vi "ziExample-HF2-ImpedanceSweep.vi"() -> ()   [LabVIEW 2009]
doc: "Control a Zurich instrument device via the LabOne Labview API. \nRequirements: Zurich Instruments HF2 (HF2IS or HF2LI-MF ).\nThis example uses the API functions to perform a frequency sweep and measure the impedance. \n\n© Zurich Instruments AG, www.zhinst.com"
uses:
  <instrlib>/Zurich Instruments LabOne/Public/Utility/Impedance/ziTypeCalib.ctl
  <instrlib>/Zurich Instruments LabOne/Public/Utility/Impedance/ziTypeCalibModel.ctl
  <instrlib>/Zurich Instruments LabOne/Public/Utility/Impedance/ziTypeImpedanceEqCircModel.ctl
  <vilib>/Utility/file.llb/Write To Spreadsheet File (DBL).vi
  <instrlib>/Zurich Instruments LabOne/Zurich Instruments LabOne.lvlib
panel:
  out "Selected Device":string
  in  "Address":string="DEV"
  out "output cluster":T1
  out "Cmd":enum16{"Idle", "Calibrate", "Measure"}(ring)
  in  "Log Sweep":bool
  in  "Voltage Gain 2":dbl=1.0 caption="Volt. Gain"
  in  "Voltage Gain":dbl=1.0 caption="Volt. Gain"
  in  "Shunt Resistor":dbl=10.0 caption="Shunt Res"
  out "cal_types":cluster{string[], bool[]}[](array[cluster])=[{["R (Ohms)", " ", " "], [TRUE, FALSE, FALSE]}, {["C (F)", " ", " "], [TRUE, FALSE, FALSE]}, {["L (H)", " ", " "], [TRUE, FALSE, FALSE]}, {["R (Ohms)", "C (F)\n ", " "], [TRUE, TRUE, FALSE]}]
  in  "PreampChannel":dbl(ring) items=["1", "2"]
  in  "Iz Demod":i32 caption="Demod"
  out "Point":i32=10 caption="Point (#)"
  in  "Iz ZCtrl":dbl(ring) items=["1", "2"]
  in  "Vz ZCtrl":dbl(ring)=1.0 caption="CA ZCtrl" items=["1", "2"]
  in  "Vz Demod":i32=3
  in  "Vz Mode":u16(ring)=1 items=["From Sig Out", "Signal Input", "HF2CA"]
  in  "Iz Mode":u16(ring)=2 items=["HF2TA", "HF2CA", "Int. Shunt", "Ext. Shunt"]
  in  "Tab Control":enum32{"Measurement", "Calibration"}(tab)
  in  "CalApply":bool
  out "Vz: Amp":T2(graph)
  out "Vz: Theta":T2(graph)
  out "C (F)":cluster{"Output":dbl[], dbl[]}(graph)={"Output"=[1000000.0, 1394950.79396242, 1945887.7175763901, 2714417.616594907, 3786479.009414645, 5281951.900505007, 7368062.997280774, 10278085.328021964, 14337423.28873774, 20000000.000000004], []}
  out "Iz (Arms)":cluster{"Output":dbl[], dbl[]}(graph)={"Output"=[1000000.0, 1394950.79396242, 1945887.7175763901, 2714417.616594907, 3786479.009414645, 5281951.900505007, 7368062.997280774, 10278085.328021964, 14337423.28873774, 20000000.000000004], []}
  out "Phase(I) (deg)":cluster{"Output":dbl[], dbl[]}(graph)={"Output"=[1000000.0, 1394950.79396242, 1945887.7175763901, 2714417.616594907, 3786479.009414645, 5281951.900505007, 7368062.997280774, 10278085.328021964, 14337423.28873774, 20000000.000000004], []}
  out "Raw Theta":cluster{dbl[], dbl[]}[](graph)=[{[1000000.0, 1394950.79396242, 1945887.7175763901, 2714417.616594907, 3786479.009414645, 5281951.900505007, 7368062.997280774, 10278085.328021964, 14337423.28873774, 20000000.000000004], [-2.125111002254364, -2.9180042427061874, -4.0042554137336674, -5.49361529933484, -7.575470258948731, -10.468749002646796, -14.656165010490133, -20.60629193272774, -29.257773273212596, -42.298319052614715]}, {[1000000.0, 1394950.79396242, 1945887.7175763901, 2714417.616594907, 3786479.009414645, 5281951.900505007, 7368062.997280774, 10278085.328021964, 14337423.28873774, 20000000.000000004], [-1.9735738261703217, -2.706927178851299, -3.6423625337918537, -4.9685737214455274, -6.862030199908028, -9.497652129209763, -13.252753090507843, -18.663185630274253, -26.628128185477088, -38.88126041886271]}, {[1000000.0, 1394950.79396242, 1945887.7175763901, 2714417.616594907, 3786479.009414645, 5281951.900505007, 7368062.997280774, 10278085.328021964, 14337423.28873774, 20000000.000000004], [0.15153717608404205, 0.21107706385488845, 0.36189287994181374, 0.5250415778893123, 0.7134400590407033, 0.9710968734370322, 1.4034119199822896, 1.9431063024534865, 2.6296450877355078, 3.4170586337520064]}]
  in  "Sweep":bool
  out "Raw Voltage":cluster{dbl[], dbl[]}[](graph)=[{[1000000.0, 1394950.79396242, 1945887.7175763901, 2714417.616594907, 3786479.009414645, 5281951.900505007, 7368062.997280774, 10278085.328021964, 14337423.28873774, 20000000.000000004], [0.023378137138417795, 0.023352635540891502, 0.02333887818292926, 0.023325702784780588, 0.023293571728526332, 0.02327435029470388, 0.023266098096908466, 0.023207676828308578, 0.023122435350856608, 0.022822802880295735]}, {[1000000.0, 1394950.79396242, 1945887.7175763901, 2714417.616594907, 3786479.009414645, 5281951.900505007, 7368062.997280774, 10278085.328021964, 14337423.28873774, 20000000.000000004], [0.011672305817526927, 0.011652162485173598, 0.01164073320249789, 0.011628802299049338, 0.011618688750611094, 0.011628538960158322, 0.011638988104010175, 0.011664869376525768, 0.011693607080250431, 0.011687890332164705]}]
  in  "SaveData":bool
  out "R (ohm)":cluster{"Output":dbl[], dbl[]}(graph)={"Output"=[1000000.0, 1394950.79396242, 1945887.7175763901, 2714417.616594907, 3786479.009414645, 5281951.900505007, 7368062.997280774, 10278085.328021964, 14337423.28873774, 20000000.000000004], []}
  out "cmp1":dbl caption="|Z| (Ohm)" format="%_5p"
  out "cmp2":dbl caption="Phi (deg)" format="%_5p"
  out "Extrapolated":bool
  in  "Unit Sel":T3=enum."|Z|, Phi"
  in  "CalibPlot":bool
  in  "Calibrate":bool
  out "Calibration Theta (deg)":T4(graph)
  in  "SaveCalib":bool
  in  "LoadCalib":bool
  in  "Calib Container":T5(array[cluster])=[{"Ref Label"="49.9", "Ref ID"=1, "Ref_Z"=[49.9+0.0i], "Meas_Z"=[100.0, 50.23729761312895, 2.121440574135451e-05, 101.32221485214248, 50.24456461049771, -2.6268567656583807e-05, 102.66191222543722, 50.24501670088856, -6.196503568242303e-05, 104.01932327637543, 50.2446244843673, -5.713301200835168e-05, 105.39468221783378, 50.24416304621723, -5.367452327358224e-05, 106.78822635948634, 50.24524269734806, -5.876089144636414e-05, 108.200196148751, 50.246354974997864, -6.364545386253118e-05, 109.63083521227709, 50.24671592753094, -6.067752029835185e-05, 111.08039039798167, 50.24580811649929, -6.479615187070807e-05, 112.54911181764163, 50.247002863074755, -5.827912157445999e-05, 114.03725289004895, 50.24804205709008, -5.481035794834855e-05, 115.54507038473645, 50.24917669390061, -5.335595986182831e-05, 117.07282446628192, 50.246949394358616, -7.292141020097264e-05, 118.6207787391978, 50.24882796722916, -6.750797590795425e-05, 120.18920029341454, 50.247846007499454, -5.7847329975082594e-05, 121.77835975036535, 50.24845718404789, -4.293736826430601e-05, 123.38853130968018, 50.248343510682076, -6.311796069229001e-05, 125.01999279649725, 50.249183273366306, -7.942521692783592e-05, 126.6730257094, 50.24772866257277, -7.427869435562275e-05, 128.34791526898795, 50.2476915178063, -7.601733111173622e-05, 130.04495046708976, 50.245533237900865, -5.583774108413694e-05, 131.76442411662694, 50.24753693734964, -7.248396684417506e-05, 133.506632902137, 50.24762342206959, -8.020141468398587e-05, 135.2718774309644, 50.24738695570386, -8.318556929612295e-05, 137.06046228512858, 50.249066459043476, -7.02076550143384e-05, 138.8726960738777, 50.24848771373767, -8.1871266738444e-05, 140.7088914869372, 50.24868744189634, -7.362994992315661e-05, 142.56936534846253, 50.25014472956201, -6.385281326676391e-05, 144.4544386717052, 50.25079362150357, -8.842270680225136e-05, 146.36443671440153, 50.24791809805706, -7.87625706591446e-05, 148.29968903489402, 50.24918621159905, -1.4247528741100358e-05, 150.26052954899453, 50.24700324146568, 2.4328293243222397e-05, 152.24729658759927, 50.24742659667306, -8.207366957398373e-05, 154.2603329550659, 50.24824371666022, -9.25027016414374e-05, 156.29998598836224, 50.24936659001939, -7.856629604557065e-05, 158.366607616997, 50.247703627076696, -8.101461803112264e-05, 160.46055442374313, 50.24847444541704, -8.360916870339348e-05, 162.58218770616404, 50.24684762067942, -8.42162391563758e-05, 164.7318735389531, 50.247774868237755, -9.143276825460823e-05, 166.90998283709771, 50.24751479542865, -9.083054064933006e-05, 169.11689141987827, 50.24687854762921, -8.032930312132663e-05, 171.3529800757136, 50.245454152632874, -0.0001002428490940411, 173.61863462786343, 50.24374595275946, -9.273543582695971e-05, 175.91424600100004, 50.24399446647822, -8.930879950739245e-05, 178.2402102886597, 50.24463642269349, -8.9468508221365e-05, 180.59692882158637, 50.24433860831839, -0.00010562198902211549, 182.98480823697858, 50.24378130866547, -9.00820622436489e-05, 185.40426054865233, 50.24277723345728, -8.794795152361801e-05, 187.85570321813157, 50.24262820801012, -9.394497153337508e-05, 190.3395592266784, 50.24087696315062, -9.303875911910995e-05, 192.8562571482761, 50.240156107300876, -0.00010294840330862538, 195.4062312235767, 50.23942030425392, -0.00010216217241291718, 197.9899214348267, 50.24028214134422, -7.679878497665776e-05, 200.60777358178322, 50.24331740451916, -4.877843237779148e-05, 203.2602393586339, 50.237629543368605, -0.00014412323110584457, 205.94777643193413, 50.237242860989426, -0.00010368709185469055, 208.67084851957435, 50.23652108204443, -0.00010531426997736317, 211.42992547079191, 50.237714097600175, -0.00011317987522256575, 214.2254833472405, 50.23871809659533, -0.00010741394236277056, 217.05800450513172, 50.23657830717324, -0.00012093921870647237, 219.9279776784627, 50.23688431881305, -0.00011039496993179517, 222.83589806334393, 50.237727239145066, -0.00011666302857080836, 225.78226740344255, 50.237920119171335, -0.0001132697762300105, 228.7675940765549, 50.23898063887997, -0.00011842913699133826, 231.79239318232413, 50.23695928588504, -0.00012264440046028195, 234.85718663111734, 50.236623190031594, -0.00012009527011622733, 237.96250323407796, 50.23849833701747, -0.0001160793104080237, 241.10887879436896, 50.23885709351022, -0.00011923738836989553, 244.29685619962234, 50.23875634780288, -0.00012605945243077108, 247.5269855156109, 50.235412702723224, -0.00014489924302107032, 250.79982408115887, 50.234219003536516, -0.00013231674153141434, 254.11593660430717, 50.235578849530135, -0.00013377463756983191, 257.4758952597503, 50.235443222241436, -0.0001349608674113157, 260.88027978756156, 50.236126095861316, -0.00013179524516250768, 264.32967759322355, 50.23542562417865, -0.00013391534137439175, 267.82468384898175, 50.23625165516228, -0.00014298573817566227, 271.3659015965364, 50.23690727788916, -0.00015680990817982095, 274.95394185109643, 50.23658453903392, -0.0001400935583827526, 278.5894237068025, 50.2379820454398, -0.00015305640734792158, 282.2729744435523, 50.23779555499338, -0.0001454244383816006, 286.005229635229, 50.23633598000316, -0.00015199925922369304, 289.7868332593705, 50.23750893219329, -0.0001422943141655904, 293.618437808279, 50.23826807223343, -0.00014498739479441598, 297.5007044016091, 50.24257243523222, -0.0002208232263127257, 301.43430290043534, 50.233676447783004, -8.696126824219892e-05, 305.4199120228374, 50.237018744070234, -0.00015812075664359103, 309.4582194610035, 50.23840482558237, -0.0001421567736495156, 313.54992199989294, 50.23720959526779, -0.00016391008918537842, 317.69572563745635, 50.238882279353724, -0.0001747339577064879, 321.89634570645694, 50.23817479484266, -0.00016711708268028609, 326.1525069978913, 50.23794493404207, -0.00016987432226198176, 330.4649438860528, 50.23942799702911, -0.00018019706189285748, 334.8344004552382, 50.239504175654254, -0.00017134177816558637, 339.2616306281399, 50.23854749803337, -0.00018134810219163985, 343.7473982959256, 50.239863616591016, -0.00018691169923698288, 348.29247745004807, 50.24004166104534, -0.00022403392716366483, 352.89765231578724, 50.24138303687455, -0.0001633680357283863, 357.5637174875691, 50.24132555893579, -0.00018109919688103212, 362.29147806606215, 50.24012695672146, -0.00019152917023744354, 367.08174979709855, 50.24048343767394, -0.00019087901930413202, 371.9353592124199, 50.23935600994191, -0.00018980468877723996, 376.8531437722964, 50.23945619593062, -0.00019207175954793134, 381.8359520100192, 50.23941024460613, -0.00019504023060529945, 386.8846436783157, 50.24004177721329, -0.00019049824526780213, 392.0000898976885, 50.23936798873412, -0.00022604853872247393, 397.183173306728, 50.23924109279576, -0.00013131812397570967, 402.4347882144, 50.23465524046287, -0.00016094847498827718, 407.7558407543593, 50.237935578787884, -0.00023442906566915965, 413.1472490412919, 50.23754191590512, -0.0002241082550303329, 418.609943329334, 50.23758477571322, -0.00020745270535459898, 424.14486617257967, 50.23844955352966, -0.00022638680937830992, 429.7529725877134, 50.23819284665975, -0.0002199711780855827, 435.4352302187919, 50.23848807847116, -0.00021746871784881117, 441.1926195042056, 50.23752737389911, -0.0002347905781568576, 447.0261338458467, 50.23723095212465, -0.00023695481260912191, 452.93677978051477, 50.237967943967085, -0.00023321305655591763, 458.9255771535886, 50.237296399116545, -0.00023583442488857333, 464.993559294994, 50.23819243539614, -0.00022819779420788495, 471.14177319749837, 50.23821404307303, -0.00023657243075930968, 477.37127969736315, 50.238454297395336, -0.0002564686351001599, 483.6831536573843, 50.23949055231677, -0.00025662562140457847, 490.0784841523534, 50.23963343470409, -0.00026991681507969946, 496.55837465697056, 50.24006446546527, -0.00019542383543565305, 503.1239432362423, 50.24006149866944, -0.00019263605772786905, 509.7763227383968, 50.241541900367416, -0.0002650210010511269, 516.5166609903497, 50.24204575422077, -0.0002680894028589533, 523.3461209957545, 50.24192028206883, -0.0002595992513746522, 530.265881135672, 50.24243515517191, -0.0002693038142289864, 537.2771353718921, 50.24194685410137, -0.00028033155549634563, 544.3810934529448, 50.243606525411785, -0.0002760762107079244, 551.5789811228353, 50.242950307895605, -0.0002691784388977296, 558.8720403325376, 50.24270972720745, -0.00028235834370080135, 566.2615294542862, 50.242641696523165, -0.0002813688997713343, 573.7487234987, 50.24297072057299, -0.0002886415178501039, 581.3349143347776, 50.24155585194577, -0.00028813043222880976, 589.0214109128019, 50.241512211068226, -0.00030399847025470696, 596.8095394901901, 50.246494416914686, -0.00030000047211699543, 604.7006438603325, 50.2411127859893, -0.00032191837745573814, 612.6960855844551, 50.24388358908722, -0.00032557214682823766, 620.7972442265484, 50.24425956315106, -0.0003281739605617717, 629.0055175914031, 50.24376088901165, -0.0003249400740398162, 637.3223219657923, 50.24400596262748, -0.00032628094469877784, 645.7490923628433, 50.243892945867564, -0.0003149332196067413, 654.2872827696401, 50.244689616316684, -0.0003224844489783764, 662.9383663980998, 50.24448603801334, -0.0003296492473939034, 671.7038359391662, 50.24385175285881, -0.00034531896154369097, 680.5852038203647, 50.2433017558709, -0.00035427140131504394, 689.5840024667617, 50.24254002402706, -0.000351718688616745, 698.7017845653758, 50.24426996580821, -0.00034292404995620675, 707.9401233330838, 50.242294710892395, -0.0003511291528132747, 717.3006127880695, 50.24320044074088, -0.000357591418540799, 726.7848680248625, 50.24384831032141, -0.0003581451947597097, 736.3945254930113, 50.24411746233949, -0.0003624322702113084, 746.1312432794441, 50.245400714741756, -0.0003768273094781495, 755.9967013945603, 50.24460116850206, -0.00038515303493329487, 765.9926020621064, 50.24386501335661, -0.0004014769252018121, 776.1206700128843, 50.24343741635483, -0.0003850526766427019, 786.3826527823423, 50.242386569716956, -0.0003944547277776726, 796.7803210121025, 50.24231847213171, -0.0004083242796739145, 807.315468755473, 50.24148533783557, -0.0004069646661488162, 817.9899137870017, 50.24304518383028, -0.0004043264799102493, 828.8054979161209, 50.24321435653486, -0.0004082179233760825, 839.7640873049413, 50.242901199777, -0.0004233529907266768, 850.867572790246, 50.24335396992659, -0.00041494558073980244, 862.1178702097428, 50.24285017263916, -0.0004250528520568761, 873.5169207326305, 50.24421089963702, -0.00044036646096422516, 885.066691194535, 50.243906111732, -0.0004455635019504344, 896.7691744368752, 50.243115112962, -0.00044548362054011836, 908.6263896507152, 50.241847736633005, -0.0004546709589164505, 920.6403827251629, 50.242469741042036, -0.000469671885646098, 932.8132266003764, 50.24200716387695, -0.0004755603159924677, 945.1470216252361, 50.242235520185325, -0.00046569926345137625, 957.6438959197473, 50.24228264021354, -0.0004560626191996769, 970.3060057422341, 50.241726115331836, -0.0004693435526159942, 983.1355358613883, 50.24250104649113, -0.000469173165346523, 996.1346999332383, 50.242280221489466, -0.0004941911752693712, 1009.3057408831005, 50.241041961032785, -0.0004972471672201722, 1022.6509312925836, 50.24065192046913, -0.0005048544802369564, 1036.1725737917075, 50.240705322833705, -0.0005120142985370826, 1049.8730014562084, 50.2409880560542, -0.0005185151977316893, 1063.7545782100965, 50.24100716912316, -0.0005256851906550238, 1077.819699233536, 50.23957008666112, -0.0005233075405538072, 1092.0707913761194, 50.24066642423129, -0.0005667882309460218, 1106.5103135756042, 50.24028373804092, -0.0005886985493355609, 1121.1407572821893, 50.23984181544734, -0.0005416423273569886, 1135.964646888397, 50.23901186463722, -0.0005469432103160592, 1150.9845401646432, 50.23992880526662, -0.000563876372453988, 1166.2030287005641, 50.239552851083815, -0.0005613410906528647, 1181.6227383521784, 50.239819261152476, -0.00055276476146632, 1197.2463296949636, 50.23718308658164, -0.00059155470497235, 1213.0764984829211, 50.23703227282794, -0.0005639536793866361, 1229.1159761137123, 50.23720604014747, -0.0005828010566710451, 1245.367530099944, 50.2376316294328, -0.000605006915033908, 1261.8339645466854, 50.23706673631338, -0.000605622450206069, 1278.5181206353, 50.23635119432776, -0.0006167725116433101, 1295.422877113673, 50.23539548733378, -0.0006297581002267215, 1312.5511507929214, 50.236467808934, -0.0006640770731730505, 1329.9058970506724, 50.23718535641903, -0.0006493956219717666, 1347.490110340995, 50.23597810259524, -0.0006575973144651183, 1365.3068247110748, 50.23612858584978, -0.0006552481232708702, 1383.3591143247195, 50.234825849623896, -0.0006571084498600002, 1401.6500939927878, 50.23411209669829, -0.0006556132494747068, 1420.1829197106294, 50.237073548758374, -0.0006957885218835113, 1438.960789202634, 50.23609605743348, -0.0006716559593610621, 1457.986942473978, 50.23655785267992, -0.0006847225644928291, 1477.2646623696671, 50.2367756747552, -0.0007089642012018262, 1496.7972751409714, 50.23461986858555, -0.0007235796678223535, 1516.5881510193492, 50.23777867946216, -0.0007067022205569458, 1536.64070479796, 50.23594013773257, -0.0007350784198242394, 1556.9583964208657, 50.23548638970917, -0.0007277415031621394, 1577.5447315800218, 50.23577058239413, -0.0007365114353948249, 1598.403262320164, 50.234764438996656, -0.0007358475139249357, 1619.5375876516912, 50.23451293620078, -0.0007669913805915337, 1640.951354171652, 50.2342973593145, -0.0007672584900687068, 1662.6482566929444, 50.234877383456855, -0.0007719410590508477, 1684.6320388818249, 50.23479457558916, -0.0007975876224606731, 1706.9064939038728, 50.23411424828983, -0.0007839190573285075, 1729.4754650784525, 50.23335239475232, -0.0008236858193597738, 1752.342846541882, 50.233956339633075, -0.0008219820643363365, 1775.5125839193133, 50.23267459889144, -0.0008248354222896179, 1798.988675005555, 50.23209385202891, -0.0008258347765294869, 1822.7751704548377, 50.23233597449878, -0.0008402376745349847, 1846.8761744797591, 50.232063575711535, -0.0008434684927485383, 1871.2958455594094, 50.23226069711804, -0.0008495184625211668, 1896.038397156923, 50.231264787120935, -0.000856226416158429, 1921.1080984464543, 50.23071209814313, -0.0008779962269724759, 1946.5092750498272, 50.23171826210217, -0.00089508111780188, 1972.246309782865, 50.22893609855841, -0.0009023291566507657, 1998.3236434116482, 50.229671960519234, -0.0009343517002818267, 2024.7457754187096, 50.228264240727206, -0.000923053626219264, 2051.517264779425, 50.22793750616886, -0.0009217625619728219, 2078.642730748604, 50.22715368622507, -0.0009448586201383313, 2106.1268536575444, 50.22981498597677, -0.0009480664328276984, 2133.9743757215633, 50.22753294140639, -0.00097696946339409, 2162.1901018582707, 50.229106040780856, -0.0009795278451825758, 2190.7789005165932, 50.22925952739951, -0.000964143533363214, 2219.74570451683, 50.22913336910716, -0.000999664726629083, 2249.095511901744, 50.22888765446308, -0.0009929226999867554, 2278.833386798981, 50.229156943383416, -0.0010356702222864209, 2308.9644602948165, 50.2275218915404, -0.001023076393648231, 2339.493931319528, 50.22746275489175, -0.0010120517700893503, 2370.427067544405, 50.2281958047674, -0.001026785817893122, 2401.769206290685, 50.22815050358506, -0.0010515565170741634, 2433.5257554504424, 50.22735832444823, -0.0010546438729483237, 2465.702194419723, 50.2270696074257, -0.0010765612187811227, 2498.3040750439413, 50.22765197797887, -0.0011118182352407738, 2531.337022575856, 50.2276471510043, -0.001101844497572114, 2564.8067366461323, 50.22721822901245, -0.0011337329910801146, 2598.718992246821, 50.22720426028747, -0.001122893143006475, 2633.0796407277535, 50.22443066210692, -0.00116261967665977, 2667.894610806198, 50.226871660032785, -0.0011483106083631292, 2703.1699095897843, 50.22526274815143, -0.0011507616972477122, 2738.9116236130294, 50.223806897500516, -0.001173247560470509, 2775.125919887495, 50.22634928448615, -0.0011913188342702536, 2811.819046965906, 50.2258071872988, -0.0011988830826533568, 2848.9973360202575, 50.22419364937601, -0.0012148498702072607, 2886.667201934264, 50.22282751934193, -0.0012123971632495361, 2924.835144410162, 50.222894099248904, -0.0012330284118999585, 2963.507749090239, 50.22246247680122, -0.001264311966019769, 3002.6916886931003, 50.221090275797124, -0.0012558228823002556, 3042.3937241650515, 50.22071885090921, -0.0012853768065090344, 3082.6207058466093, 50.221689332713005, -0.0012939793355571283, 3123.379574654536, 50.219118508740856, -0.0012900490004014427, 3164.6773632793997, 50.22018200020054, -0.001321423076319436, 3206.521197399074, 50.219804467487094, -0.0013217581465878262, 3248.9182969081785, 50.21896416346328, -0.0013519130644718818, 3291.8759771638765, 50.21723415283566, -0.0013394520641220394, 3335.401650248044, 50.21907848822479, -0.0013708606750503596, 3379.502826246233, 50.217898207990075, -0.001378802620359021, 3424.187114543432, 50.21712744965305, -0.0013947676225755856, 3469.462225137078, 50.21626045719793, -0.0014316210807793785, 3515.3359699673097, 50.21657172729146, -0.0014384263510618701, 3561.816264264928, 50.21680400626807, -0.0014298789475400897, 3608.911127917062, 50.21542751168883, -0.0014498958934021917, 3656.628686851008, 50.21531737343841, -0.0014561937888761822, 3704.9771744362506, 50.21600817244085, -0.001479176684521728, 3753.9649329051394, 50.21546053357334, -0.0014933670389546691, 3803.600414792228, 50.2158560392781, -0.0014998415604633158, 3853.892184392768, 50.213392846741534, -0.0014985775764123394, 3904.848919240363, 50.21376680888128, -0.0015172310065091246, 3956.4794116042885, 50.20971735456384, -0.001548487872186491, 4008.7925700064757, 50.21014702413487, -0.001587379265308434, 4061.79742075869, 50.21210668637432, -0.001569131703590054, 4115.503109519897, 50.212328610000554, -0.001591197976474863, 4169.918902874359, 50.20953605449185, -0.001610756285018924, 4225.054189930457, 50.209195201621384, -0.0016196734346381205, 4280.91848394079, 50.209152833782134, -0.0016462892603500098, 4337.521423943564, 50.20929118358185, -0.0016251392376527788, 4394.872776425812, 50.21095848686051, -0.0016629976090468473, 4452.982437008476, 50.20839299137227, -0.0016816139048923943, 4511.860432153903, 50.20949627211689, -0.0017025116900396776, 4571.516920895777, 50.207208132836705, -0.0017019845210760162, 4631.962196592072, 50.20624686545255, -0.0017375850579768393, 4693.206688701033, 50.206960888920555, -0.0017450280831560023, 4755.260964580788, 50.205874125136766, -0.0017706140596811606, 4818.135731312604, 50.2053796616479, -0.0017860174631342419, 4881.841837548408, 50.203669761043294, -0.0017986881613215938, 4946.390275382573, 50.204084313435814, -0.0017930213428036259, 5011.792182248618, 50.20102117012197, -0.0018024389465272194, 5078.0588428408255, 50.20227458721212, -0.0018411233943555132, 5145.201691061401, 50.20196042844434, -0.0018547169024248672, 5213.232311993302, 50.199039599936306, -0.0018657872889419546, 5282.162443899168, 50.198885905963316, -0.0018629462681835364, 5352.0039802466945, 50.1989062406597, -0.0019250037187925912, 5422.768971760774, 50.19873078080312, -0.0019318836231305252, 5494.4696285027685, 50.19617164427985, -0.0019494800265833334, 5567.11832197729, 50.20026970728898, -0.0019544295196609156, 5640.727587266819, 50.197179048361754, -0.001960458372925354, 5715.310125194559, 50.19649143154678, -0.0019908171741621016, 5790.878804515884, 50.195813741075284, -0.0020115561068027314, 5867.446664138765, 50.19462655684263, -0.002032850682276669, 5945.026915373546, 50.19513569207532, -0.002048686109170098, 6023.632944212483, 50.193531233283984, -0.0020719039867506065, 6103.278313639408, 50.19219200595069, -0.002058353012787509, 6183.97676596994, 50.191926195949335, -0.002097465747676496, 6265.742225222635, 50.19018269513743, -0.0021363159051956816, 6348.588799521492, 50.191582144458366, -0.0021285438857643127, 6432.530783530218, 50.188361574893804, -0.0021611951311052316, 6517.582660918692, 50.18689112272658, -0.0021951638367680884, 6603.759106862022, 50.18645598993114, -0.002182507086802017, 6691.074990572664, 50.18653648884716, -0.0022380354802923135, 6779.545377866007, 50.1841298541305, -0.002232150619787658, 6869.185533759891, 50.185273542271574, -0.0022552517710957595, 6960.010925108487, 50.18223849352442, -0.002299632550290506, 7052.037223271011, 50.18230204881788, -0.002295428510750354, 7145.280306815716, 50.181784637314614, -0.0023034341643105617, 7239.756264259645, 50.179442819860334, -0.0022999160910138917, 7335.481396844602, 50.18049666351586, -0.002336220384334037, 7432.47222134983, 50.17748051325628, -0.002376214418226106, 7530.745472941882, 50.176382193509674, -0.0023931312387562927, 7630.318108062167, 50.174775680856634, -0.0024154919127549416, 7731.207307352683, 50.17465021843281, -0.0024205294729742937, 7833.430478620425, 50.17272069027671, -0.0024788396977582106, 7937.005259840999, 50.172347060671655, -0.002485901661517948, 8041.949522201948, 50.1698419603063, -0.002472246110630353, 8148.281373186303, 50.16654372906631, -0.002490807597431718, 8256.019159696933, 50.166546637917385, -0.0025278093779786607, 8365.181471222173, 50.165666710672745, -0.0025458956999909904, 8475.787143043344, 50.15924317939559, -0.002559511896967234, 8587.855259484646, 50.160873766543894, -0.0025874125237846848, 8701.40515720605, 50.16103150912793, -0.00259330692047426, 8816.456428539721, 50.15877184751908, -0.0026368428148966327, 8933.028924870545, 50.1583599738148, -0.0026157253223961343, 9051.142760061368, 50.15391746682331, -0.002649629721455793, 9170.818313923517, 50.15639620269551, -0.0026419954711127164, 9292.076235733217, 50.15600457102218, -0.002690759557057573, 9414.937447794484, 50.152270092909085, -0.002711539596102655, 9539.423149049147, 50.151229918303926, -0.002733239806867122, 9665.554818734592, 50.14817335051223, -0.0027283481453376736, 9793.354220089876, 50.14838501435081, -0.002777513245041367, 9922.843404110825, 50.14498409143958, -0.0028080804496252183, 10054.04471335481, 50.143191824712254, -0.002798653022874521, 10186.980785795844, 50.14131333919284, -0.0028376181480733345, 10321.674558730547, 50.142351836679175, -0.002806299037077858, 10458.149272735884, 50.14014039134109, -0.002841401486001693, 10596.428475679219, 50.135756344174034, -0.0028778563196009336, 10736.536026781316, 50.1327191062114, -0.002877300971482413, 10878.496100733057, 50.13296037178068, -0.00289226158486279, 11022.333191866679, 50.133420784302935, -0.00290040547989766, 11168.072118382159, 50.13032843275592, -0.00292132250458899, 11315.738026629404, 50.13010470676568, -0.002963285670636231, 11465.356395447043, 50.12725730425856, -0.002947550707445533, 11616.953040558701, 50.12473033832046, -0.0029702000623227118, 11770.554119027373, 50.125358324481375, -0.002978072835499054, 11926.186133768635, 50.123322964124085, -0.003026178469715618, 12083.875938123492, 50.12148744546602, -0.003025221810037537, 12243.650740491821, 50.11528210759404, -0.003020030098309541, 12405.538109027044, 50.11457700524859, -0.0030507319222068023, 12569.565976392809, 50.11284714955164, -0.0030687506775841406, 12735.762644582535, 50.111906869623546, -0.003044497075707217, 12904.156789802806, 50.11038768487796, -0.003052387418891352, 13074.777467421318, 50.10934188694288, -0.0030933862369993907, 13247.654116980155, 50.10784795385326, -0.0030730577874665977, 13422.816567275346, 50.104553702134666, -0.003151006860357638, 13600.295041503688, 50.10407101352109, -0.003118305371306654, 13780.120162477633, 50.10100484356877, -0.003145179358625191, 13962.322957909008, 50.096177561991155, -0.003131377703532754, 14146.934865762594, 50.09881326561069, -0.0031161878643231997, 14333.987739680617, 50.09537711463793, -0.003155950060110272, 14523.51385447894, 50.09281302426684, -0.0031645457509371917, 14715.545911715848, 50.089610730638604, -0.0031278585028689855, 14910.117045334415, 50.088456909798595, -0.0031300262894056094, 15107.26082737964, 50.08674511388334, -0.003175790287680866, 15307.01127379114, 50.085150571481215, -0.003198688651147788, 15509.402850272347, 50.08269308396382, -0.0032208223997844433, 15714.470478237274, 50.08079653546898, -0.003174994452040102, 15922.249540836057, 50.07910740339394, -0.003208284255155545, 16132.775889060164, 50.07739263436712, -0.0031814151108409783, 16346.085847928194, 50.072219822234416, -0.0032278686717667044, 16562.21622275348, 50.070003460994705, -0.0031892459930366033, 16781.20430549466, 50.06369746665929, -0.0032199579581452488, 17003.087881190266, 50.06379797457856, -0.0032478656244064904, 17227.90523447822, 50.06591198969062, -0.0032168021156868416, 17455.695156201542, 50.0607304586169, -0.0032256520442505315, 17686.496950101537, 50.06057965910033, -0.0032075235196186, 17920.350439599486, 50.057000186074355, -0.003221606255168424, 18157.29597466787, 50.05065362984461, -0.0032378838277122147, 18397.374438792416, 50.04745857976109, -0.003206821686866474, 18640.627256026375, 50.04682482941959, -0.003218824549749692, 18887.096398138056, 50.04508507521049, -0.003231834976687231, 19136.824391852726, 50.04300107978831, -0.00323229619365187, 19389.85432619025, 50.040496822637465, -0.00320470848620476, 19646.229859899908, 50.03768941842796, -0.0032553646796862493, 19905.995228993535, 50.03909512882343, -0.0032285610303332954, 20169.195254378083, 50.03609384577493, -0.0031889148984652373, 20435.875349589107, 50.030830423780266, -0.0031795383763224346, 20706.081528626677, 50.027689884726705, -0.003198047205025663, 20979.860413894887, 50.02636488232802, -0.0032039233746700728, 21257.25924424619, 50.02515579276422, -0.0032039473709047986, 21538.325883132064, 50.01920781261719, -0.0032067642841510386, 21823.108826861662, 50.01782122657808, -0.0031882922254780816, 22111.65721296962, 50.01477815340255, -0.0031519388487804426, 22404.020828694363, 50.01637100655501, -0.0031786768132729534, 22700.250119568478, 50.01043774454449, -0.0031431569785494995, 23000.396198122882, 50.01262465065033, -0.0031875200185355833, 23304.510852706055, 50.005923169030346, -0.0031228449073645655, 23612.646556419713, 50.00977985357827, -0.003083156085068887, 23924.85647617263, 50.00197891498816, -0.003099346539094118, 24241.194481854334, 50.00154611416805, -0.003108041981316244, 24561.71515563013, 49.996372839552464, -0.0030435152301369604, 24886.47380135883, 49.996734467785295, -0.0030382637795891006, 25215.526454134968, 49.99271499415384, -0.0030690162111026422, 25548.92988995743, 49.99112419924288, -0.0030438735768337664, 25886.74163552589, 49.990891448575496, -0.003064664453722693, 26229.019978166594, 49.98561479733623, -0.003010781321876719, 26575.823975889358, 49.98349848762823, -0.0029523930266150363, 26927.21346757778, 49.98221735168488, -0.0029699550875510084, 27283.249083314236, 49.97825100196772, -0.00297747605964099, 27643.992254840872, 49.97699569495667, -0.0029303048187205947, 28009.50522615947, 49.97198369208348, -0.002945362838796895, 28379.851064271345, 49.97178787770749, -0.002900468286124499, 28755.093670059083, 49.96834679642961, -0.00289619025926756, 29135.297789312117, 49.962990467014926, -0.0028928572884370555, 29520.529023898314, 49.96403104512659, -0.0028451833794340135, 29910.8538430833, 49.96388114787904, -0.0028232001635142595, 30306.33959499921, 49.953610534815105, -0.002813660364559434, 30707.054518265057, 49.95001704032324, -0.002778198326570019, 31113.067753761014, 49.9564081143517, -0.0027591682190586794, 31524.44935655836, 49.95156043068512, -0.002745218911362265, 31941.270308006944, 49.94817882586275, -0.0026927823101291276, 32363.602527982424, 49.94762928051548, -0.00272150122541467, 32791.51888729574, 49.9405861056004, -0.0026395381440130128, 33225.09322026663, 49.94015542002195, -0.0026394451988899594, 33664.400337463216, 49.937848467122684, -0.0025892960516466497, 34109.516038609894, 49.936097115806135, -0.0026106099535650015, 34560.51712566628, 49.93137413940305, -0.002569612346604735, 35017.48141607905, 49.9247155855568, -0.002479043005889313, 35480.48775620872, 49.924232143499744, -0.002527716901959055, 35949.61603493394, 49.919868514670505, -0.002443439526019186, 36424.947197436, 49.920121009968746, -0.0023653185663999455, 36906.563259165516, 49.91926341820065, -0.0024149936408989258, 37394.547319993595, 49.916501572239916, -0.002392160181777546, 37888.98357855004, 49.91193812300948, -0.0023455917056051214, 38389.95734675142, 49.90959033493756, -0.002335296180901407, 38897.555064521286, 49.90603746897938, -0.0022206827250308603, 39411.864314704726, 49.90421319674217, -0.002222931478725969, 39932.97383818004, 49.901204067684596, -0.002215698981253079, 40460.97354917059, 49.89896392755565, -0.0021712642328330714, 40995.95455075912, 49.89417416440868, -0.0020939896581843274, 41538.00915060688, 49.89195280794883, -0.002075562600979887, 42087.23087688055, 49.89215360169899, -0.002030482913679642, 42643.71449439012, 49.887581903887074, -0.001966593521394562, 43207.55602094014, 49.88324059638469, -0.0019395897314145418, 43778.85274389684, 49.8814218039801, -0.001896155863909438, 44357.703236974274, 49.8761371638703, -0.0018441287055229103, 44944.20737724279, 49.87491191955499, -0.001863936888100369, 45538.466362362364, 49.87106416978853, -0.0017347260644060604, 46140.582728043475, 49.86515774682025, -0.0017213875432891428, 46750.6603657388, 49.86521537157402, -0.0016818451163385347, 47368.80454056924, 49.86179102265859, -0.0016885576921970627, 47995.12190948694, 49.85789940391005, -0.0016587887833956426, 48629.720539678114, 49.855332368231615, -0.0015466322543901886, 49272.70992720917, 49.85548318566192, -0.00146059663339112, 49924.20101591977, 49.84478419997218, -0.001446260945395411, 50584.306216565674, 49.84182439253915, -0.0014136734616786901, 51253.13942621439, 49.84294638019854, -0.0013546012046470348, 51930.81604789714, 49.840997504121844, -0.0013119461168156306, 52617.453010521174, 49.835544385306164, -0.0011614975240850339, 53313.168789045325, 49.83052923638645, -0.0011180751728694885, 54018.083424921926, 49.83103446013695, -0.001079983213959617, 54732.318546809016, 49.824198434903806, -0.0008938238493060074, 55455.997391556804, 49.81929289056292, -0.0008986713162491293, 56189.24482547166, 49.81979542727113, -0.0007335091334085476, 56932.18736586081, 49.811071849464696, -0.0006879118009670016, 57684.95320286186, 49.80594074138474, -0.0006715967324208361, 58447.67222156148, 49.804215535907524, -0.0004772957409515872, 59220.47602440647, 49.79832579549923, -0.0004842269726905048, 60003.49795391071, 49.792280020704936, -0.000307746097213962, 60796.87311566238, 49.790350069282994, -0.000169852049503953, 61600.738401635834, 49.787236168034134, -0.0001615806220574499, 62415.232513811636, 49.77994516866089, 0.00011060975733758773, 63240.49598810858, 49.77823198455395, 0.0003158480492937976, 64076.671218631986, 49.7775595565574, 0.0002893359567063388, 64923.90248224318, 49.77606069387036, 0.0006391000583581558, 65782.33596345384, 49.769192697525874, 0.0008772174284374898, 66652.11977964896, 49.77041559909556, 0.0012305725780833395, 67533.40400664334, 49.772421474847235, 0.0015869268152327602, 68426.34070457649, 49.78277604805913, 0.002495654925651838, 69331.08394414996, 49.92603526105637, 0.0035931804079403214, 70247.78983321095, 49.96361527664381, 0.0010075108216106457, 71176.61654368757, 49.93920885035811, -0.001039429460098497, 72117.72433888064, 49.87769822462116, -0.0026866377211722235, 73071.27560111642, 49.70569634771859, 0.00019070657642270589, 74037.43485976441, 49.72815159729473, 0.0003300894506538251, 75016.36881962561, 49.749635521994236, 0.0006272065770804981, 76008.24638969661, 49.745770827484044, 0.0010263135740020864, 77013.23871231415, 49.75175163056408, 0.0011987776738266566, 78031.5191926844, 49.75107112481251, 0.0013737909933407763, 79063.26352880256, 49.7497898892403, 0.0014320488621712344, 80108.64974176885, 49.74897198837285, 0.0015110306434432924, 81167.85820650525, 49.75782904233533, 0.0016869873599791466, 82241.0716828777, 49.75712456161475, 0.0017767899990833106, 83328.47534722992, 49.75306420869283, 0.0019190449775075913, 84430.2568243348, 49.752879222801724, 0.0020169871991360436, 85546.60621976812, 49.74852832789275, 0.0020692581556178923, 86677.71615270982, 49.748498504959045, 0.0022260616785250457, 87823.78178917895, 49.74661448992254, 0.002331258505076117, 88985.00087570857, 49.74673626293629, 0.0024571045405144686, 90161.57377346623, 49.743902877101476, 0.002494797388802399, 91353.70349282448, 49.742627740668524, 0.002703717692190503, 92561.59572838891, 49.74590197812264, 0.002724910836371634, 93785.45889448965, 49.73794384980248, 0.0027931640566752004, 95025.50416114248, 49.74039008669453, 0.0029431676795485286, 96281.94549048448, 49.73556554340275, 0.0030477668815732267, 97554.99967369149, 49.7356247392358, 0.0032139935957324144, 98844.8863683845, 49.73356392122428, 0.0032256583353969855, 100151.82813653053, 49.73024729416789, 0.0034093087571856946, 101476.05048284406, 49.72628363711887, 0.0034959230795028767, 102817.78189369592, 49.72772793495911, 0.003645172350885068, 104177.25387653774, 49.72931431253726, 0.0037215044804755613, 105554.7009998474, 49.72206489153405, 0.0038790182349691983, 106950.36093360207, 49.724915847841785, 0.003957656106730743, 108364.47449028626, 49.718209607965996, 0.004108385077346477, 109797.28566644287, 49.718851602221086, 0.004207971433699482, 111249.04168477377, 49.71594846464826, 0.00436306653103642, 112719.99303679614, 49.713294902979605, 0.004455066182347376, 114210.39352606275, 49.717703217990014, 0.004651783156347022, 115720.5003119546, 49.71764959803388, 0.004778994675681682, 117250.57395405274, 49.71061488032396, 0.004905259742818935, 118800.87845709565, 49.709258847668885, 0.005005885141156695, 120371.68131653123, 49.70797258940799, 0.005192155347462448, 121963.2535646719, 49.70813996009755, 0.005300247185998274, 123575.86981746006, 49.70509904176744, 0.005469700830152211, 125209.8083218509, 49.70264585440807, 0.005588377037671833, 126865.35100382168, 49.698738028572464, 0.0056959395789260925, 128542.78351701677, 49.69701474897347, 0.005854557359894955, 130242.39529203599, 49.698194206776364, 0.006095166085923106, 131964.47958637355, 49.70353289576618, 0.0061808802071798095, 133709.33353501724, 49.699043223231875, 0.006267658294239524, 135477.25820171784, 49.696603889129314, 0.0066786073866889045, 137268.55863093623, 49.702884935659284, 0.006862609071249372, 139083.54390047654, 49.69677159507001, 0.006821836003712494, 140922.52717481487, 49.729595860443, 0.005956444071163939, 142785.82575913466, 49.678256405756976, 0.006225137993025695, 144673.76115407608, 49.67657194253595, 0.007464824466257912, 146586.65911120857, 49.68205692115046, 0.007448449096385059, 148524.84968923658, 49.68106537450013, 0.007634100383033603, 150488.66731094982, 49.68715817052267, 0.007618440238686416, 152478.45082092631, 49.68452630295357, 0.007819218891202948, 154494.54354399754, 49.68035309321481, 0.008048182023418183, 156537.29334448618, 49.683552463511084, 0.008198403273637224, 158607.05268622865, 49.675106514761794, 0.008362708290957288, 160704.17869339127, 49.6770805590082, 0.008535179418475163, 162829.03321208904, 49.67253655290357, 0.008733796542899214, 164981.98287281947, 49.67676570766077, 0.008955204880007067, 167163.3991537229, 49.67346412094591, 0.00903903204465555, 169373.65844467946, 49.6750605037161, 0.009239440326578282, 171613.14211225224, 49.67597466720505, 0.009401071142264163, 173882.23656548903, 49.676852627858004, 0.009663675496760284, 176181.33332259525, 49.66744404430506, 0.009823648681837759, 178510.8290784891, 49.666850612236956, 0.010030277838985791, 180871.12577324774, 49.6739739271621, 0.010101540554500703, 183262.63066145912, 49.666216258196556, 0.010483543231883096, 185685.75638249176, 49.66675983225166, 0.010595849253695026, 188140.921031694, 49.67152342163504, 0.010692295736064776, 190628.5482325329, 49.66299954793407, 0.01095342929749596, 193149.06720968723, 49.662024605031434, 0.011117550036012482, 195702.91286310818, 49.665828136261794, 0.011357138581537885, 198290.52584305947, 49.65971777438311, 0.011560204492025638, 200912.35262614803, 49.66369933374925, 0.011809879686839624, 203568.84559236004, 49.659230980442686, 0.011990749836858576, 206260.463103117, 49.664212932244716, 0.012205975739571048, 208987.66958036408, 49.66735703215869, 0.012624841158656067, 211750.9355867023, 49.67109257341583, 0.012269162510871606, 214550.7379065806, 49.65746729451884, 0.012589546273321485, 217387.55962856245, 49.657267176439184, 0.013063596504474083, 220261.89022868118, 49.65895989932838, 0.013265254405043194, 223174.2256548948, 49.661536329578084, 0.013519192291749053, 226125.06841265803, 49.657920262890926, 0.013813472633583814, 229114.9276516273, 49.654921864968024, 0.013927705941009115, 232144.3192535124, 49.657723232536156, 0.014151551819086935, 235213.76592108764, 49.65721159663454, 0.014478039050487961, 238323.79726838015, 49.65561446575389, 0.014769011385865512, 241474.94991205237, 49.6484312636851, 0.014869857920882761, 244667.76756399288, 49.65207149431387, 0.015226995203148524, 247902.8011251297, 49.65120493089856, 0.01544061664088752, 251180.60878048366, 49.65675338797609, 0.015661212592290474, 254501.75609548087, 49.65121178203188, 0.015800915448757172, 257866.816113539, 49.65226073103706, 0.016244122743742588, 261276.36945493944, 49.652183791969435, 0.016416911392511394, 264731.00441701105, 49.65203713013424, 0.016667935858144627, 268231.31707563845, 49.652441763431796, 0.016927895874419986, 271777.9113881102, 49.64950884265619, 0.01711395883859534, 275371.39929732674, 49.64334945218329, 0.017473533403027944, 279012.4008373883, 49.654813744110704, 0.017797714235827714, 282701.54424057924, 49.64955003433717, 0.01792602309350117, 286439.4660457646, 49.65018178334262, 0.018243906356328627, 290226.8112082197, 49.64951669695504, 0.01860608679201045, 294064.23321091395, 49.642364763435495, 0.018755840674167915, 297952.39417726727, 49.64777787884335, 0.01922706896230094, 301891.9649853935, 49.64192471056538, 0.019447393170520844, 305883.6253838555, 49.645447133948316, 0.0197472303575397, 309928.06410895236, 49.644116032880405, 0.019982579532083655, 314025.9790035583, 49.645171317278454, 0.02035896638238244, 318178.0771375295, 49.645595995701825, 0.020606310452769297, 322385.0749297036, 49.642856031707545, 0.020959220725991174, 326647.6982715145, 49.64514323337898, 0.02126502493223368, 330966.68265224167, 49.64367493245144, 0.021471578641861964, 335342.7732859132, 49.64806899557867, 0.02194000219086832, 339776.72523988644, 49.64585536222392, 0.022280143382324195, 344269.3035651312, 49.64173753858422, 0.022608868763354762, 348821.2834282365, 49.646215676624216, 0.022954102029731766, 353433.45024515904, 49.63834886278874, 0.023314641006158265, 358106.5998167405, 49.64841566057893, 0.02352091393443067, 362841.5384660195, 49.64135220466091, 0.023878136275129046, 367639.08317735913, 49.636955053942316, 0.02436539763875636, 372500.061737411, 49.641585717751134, 0.024672952146738314, 377425.31287794333, 49.63489478516549, 0.024936084868814906, 382415.68642056035, 49.63776496711303, 0.02526821078481262, 387472.04342333524, 49.63751739448121, 0.025718150829405463, 392595.2563293789, 49.64121616606825, 0.02622186493260189, 397786.2091173733, 49.63690512830883, 0.026353380191766525, 403045.7974540973, 49.635905112842856, 0.02677840475117155, 408374.9288489711, 49.63201547713029, 0.027215761631630843, 413774.5228106389, 49.631591991639155, 0.027547272888183084, 419245.51100562327, 49.640072641875165, 0.02802792128958419, 424788.83741907985, 49.637515027121744, 0.028481256978191545, 430405.45851767785, 49.6451477450106, 0.028934404806733923, 436096.343414631, 49.638046131311384, 0.029338081102273733, 441862.47403691, 49.63977164466293, 0.029591524549592615, 447704.84529466974, 49.63781873621942, 0.030057399047405148, 453624.4652529169, 49.63158461807294, 0.030489551736137335, 459622.3553054434, 49.63613345797455, 0.030792808874662483, 465699.55035105953, 49.632231265613754, 0.03137927414633902, 471857.09897216153, 49.62828542082507, 0.03176477078164524, 478096.0636156596, 49.632044422188635, 0.032238386664439435, 484417.5207762949, 49.6367453797931, 0.032613467832733285, 490822.56118237996, 49.63990129172991, 0.033095375861897834, 497312.28998399904, 49.63234993427242, 0.03359251081669976, 503887.8269436968, 49.63054191880685, 0.03400198872443786, 510550.3066296849, 49.632289149691445, 0.034584152604917366, 517300.8786116021, 49.62798836923148, 0.03510842841966697, 524140.70765886776, 49.632951980489146, 0.035421572223046115, 531070.9739416575, 49.635205273544486, 0.03598574975435096, 538092.8732345323, 49.63429952529513, 0.03644478982896454, 545207.6171227602, 49.63173013565619, 0.03697756426398462, 552416.4332113689, 49.63247153127305, 0.037483293694130976, 559720.5653369647, 49.636068140900505, 0.03815253015820991, 567121.2737823465, 49.63136010101898, 0.03856385034960235, 574619.8354939569, 49.64089547538851, 0.03896996562667114, 582217.544302214, 49.633489066263905, 0.03973095555813413, 589915.7111447566, 49.63460915922049, 0.040209519283317514, 597715.6642926352, 49.63022069237258, 0.0406244450259222, 605618.749579495, 49.629016411842, 0.04120940248367652, 613626.3306337942, 49.633361904928506, 0.04187319744892036, 621739.7891140905, 49.62601938383967, 0.0423866659500722, 629960.524947437, 49.630223811459906, 0.04298249203850107, 638289.9565709274, 49.62346114515538, 0.04344050359971239, 646729.5211764413, 49.630423851816346, 0.0442166180679108, 655280.6749586255, 49.63254343375441, 0.04451233444716405, 663944.8933661486, 49.621870362031636, 0.0453787860203368, 672723.6713562781, 49.62447617672375, 0.04600521564960333, 681618.5236528283, 49.62417557270914, 0.046629067559239464, 690630.9850075196, 49.61800764752947, 0.0473248716569726, 699762.6104647877, 49.6245307179635, 0.04778068698028719, 709014.9756300937, 49.61603453199361, 0.0485119155638049, 718389.6769417885, 49.621173516009115, 0.049272624703494236, 727888.3319465705, 49.624686667105536, 0.04992148881254933, 737512.579578581, 49.62198801034061, 0.05041807445060276, 747264.0804421889, 49.62253579289751, 0.05127133180082281, 757144.5170985206, 49.62365227076617, 0.05181452490567133, 767155.594355779, 49.62643411531398, 0.05272551696342637, 777299.0395633939, 49.61936700863144, 0.053190673458333684, 787576.6029100628, 49.62882328759233, 0.053795169004209144, 797990.057725738, 49.62523241714513, 0.05489546857245544, 808541.2007876072, 49.62498414621174, 0.05535293822274542, 819231.852630113, 49.62438025329984, 0.056106374293436054, 830063.8578590712, 49.62458644356495, 0.05698805625479531, 841039.0854699499, 49.6181709137518, 0.0577552505070258, 852159.429170356, 49.61822551792226, 0.05852167310449932, 863426.8077067799, 49.62506345468921, 0.05920456885912213, 874843.1651956595, 49.61217629046524, 0.06009430308095894, 886410.471458829, 49.61624169902126, 0.060932818838929495, 898130.722363403, 49.61662838886595, 0.061758634739954105, 910005.9401661474, 49.619455436099166, 0.062408377690662355, 922038.173862404, 49.612266167129725, 0.06330180152249114, 934229.499539635, 49.62081083728092, 0.0642799167655366, 946582.0207356435, 49.60590687583977, 0.06517074641048902, 959097.8688015216, 49.606715375823455, 0.0659589670133454, 971779.2032693983, 49.62658367888714, 0.0667904268924677, 984628.2122250572, 49.604750194280065, 0.06780535853198685, 997647.1126854809, 49.6049059311779, 0.06860680597493862, 1010838.15098138, 49.60859429758189, 0.06941739375697673, 1024203.6031447793, 49.60054494679609, 0.07029646281838103, 1037745.7753017369, 49.596780386901486, 0.07138866748457015, 1051467.0040702587, 49.60377142954872, 0.07236435189549513, 1065369.6569634522, 49.61175236996207, 0.07362378082703641, 1079456.1327980435, 49.60465224296899, 0.07413149146976279, 1093728.862108261, 49.610310048354776, 0.07514670187035177, 1108190.3075652265, 49.610191724631804, 0.07612142915855444, 1122842.9644018563, 49.61022499002604, 0.07731019410558274, 1137689.3608434156, 49.60500812440567, 0.07819949689549258, 1152732.058543731, 49.60050711858944, 0.07947372626278099, 1167973.6530272053, 49.599355895264594, 0.08022293671485703, 1183416.7741366408, 49.59597168038136, 0.08164480043840583, 1199064.0864870222, 49.58083841082307, 0.08293641396445697, 1214918.2899252588, 49.59913043399823, 0.08371920854200936, 1230982.1199960473, 49.58604416590769, 0.08467825091753853, 1247258.3484138523, 49.585258706485895, 0.08582992664786078, 1263749.7835411686, 49.58947059168066, 0.08676713039569821, 1280459.270873067, 49.588629374128985, 0.08814121380286244, 1297389.6935281875, 49.595362217612134, 0.0892940648231091, 1314543.9727461815, 49.582810007466165, 0.09042743376785974, 1331925.0683917769, 49.57209356101321, 0.0917122774602094, 1349535.9794654604, 49.575429429903906, 0.09305859136129106, 1367379.7446209607, 49.59175224174902, 0.09408867098572227, 1385459.4426895254, 49.581745448382065, 0.09539137494858081, 1403778.1932111783, 49.58272787734322, 0.09655381143925669, 1422339.1569729524, 49.5779938617059, 0.09803370807244666, 1441145.5365542884, 49.56019909860808, 0.09927722756389018, 1460200.5768795963, 49.56660456928806, 0.10072761062513796, 1479507.56577817, 49.56174630951841, 0.10180874894195518, 1499069.8345514592, 49.57025951231637, 0.10345827580648591, 1518890.758547888, 49.548271338340754, 0.10461132882042183, 1538973.757745226, 49.56200436982151, 0.10599567823895685, 1559322.2973407102, 49.55470638217916, 0.10748709775665893, 1579939.8883489168, 49.55583218763649, 0.10855340968359734, 1600830.0882075913, 49.5550373852037, 0.1104367937590876, 1621996.501391436, 49.55683161929024, 0.11193513497651723, 1643442.7800340666, 49.55063144424771, 0.11330489214022191, 1665172.6245581387, 49.538244372024124, 0.11478831178609841, 1687189.784313859, 49.54107503381041, 0.11626824276870734, 1709498.0582258857, 49.54930133526043, 0.11770798661565814, 1732101.2954488376, 49.531386405267895, 0.11956292828896874, 1755003.3960314125, 49.530171173285886, 0.12099584992322145, 1778208.3115893467, 49.5171161070402, 0.12257447338489658, 1801720.0459872112, 49.54352859170191, 0.12401385751087124, 1825542.6560292845, 49.54167129327835, 0.12586922856122673, 1849680.252159498, 49.52071075227777, 0.12756923091373903, 1874136.9991706994, 49.530257930115745, 0.1289712186897754, 1898917.1169232298, 49.521914669947286, 0.13081252520385936, 1924024.8810730665, 49.50393588497849, 0.13250261729893195, 1949464.6238095295, 49.509631270335234, 0.134120085322027, 1975240.7346028045, 49.51468311673572, 0.13607448842869835, 2001357.6609612892, 49.496392624624065, 0.13813743669444714, 2027819.9091990127, 49.506663313663005, 0.1398099062383817, 2054632.0452131422, 49.49305595736022, 0.14155376653685262, 2081798.6952718312, 49.502373333018795, 0.14319708181107538, 2109324.5468124216, 49.48127746643555, 0.14552580443304386, 2137214.349250265, 49.485895731510816, 0.1471135428993691, 2165472.91479817, 49.475960464296534, 0.14917712247430173, 2194105.119296756, 49.47809357248287, 0.15113901941237964, 2223115.9030557144, 49.465975121550386, 0.15320625866258278, 2252510.2717062607, 49.45108138518886, 0.15551999159003807, 2282293.2970647938, 49.45536390280404, 0.15717037997686636, 2312470.118008039, 49.4537572456381, 0.15906228469140413, 2343045.9413596955, 49.4512639668443, 0.16163159047288436, 2374026.0427888776, 49.43952960825039, 0.16370594392871357, 2405415.7677203603, 49.432066233217, 0.16570515234291136, 2437220.5322569385, 49.430961894463316, 0.1677062977718995, 2469445.824113903, 49.416594842349, 0.17026981900539975, 2502097.203565952, 49.395978938209474, 0.1724676127448896, 2535180.30440654, 49.40915292792351, 0.174591348526493, 2568700.834919997, 49.38680628778157, 0.1769421737293928, 2602664.5788664147, 49.377456925420994, 0.17923664232058042, 2637077.3964796406, 49.39546494983998, 0.18155561215506763, 2671945.225478384, 49.36881390785843, 0.1839589127625186, 2707274.082090774, 49.36516177840667, 0.18626734178268975, 2743070.062092379, 49.34638673068356, 0.18893590102650878, 2779339.3418580415, 49.33598934047468, 0.19126905948206122, 2816088.179427525, 49.35084707926762, 0.1939764232661262, 2853322.9155853475, 49.343281848448875, 0.19652994935907292, 2891049.974954799, 49.34482671610089, 0.19929192074773228, 2929275.8671065154, 49.30868840459157, 0.20184402822057096, 2968007.1876816205, 49.30269699053073, 0.20456625504029857, 3007250.6195298065, 49.2951871987795, 0.20697110916816402, 3047012.9338623732, 49.276036752969404, 0.20994995863026197, 3087300.991420607, 49.28755657722973, 0.21275265819308475, 3128121.7436595093, 49.270953930379626, 0.21542203980897517, 3169482.2339472766, 49.25466445477979, 0.21838467512227347, 3211389.5987805417, 49.262914947138384, 0.22106993629718133, 3253851.0690157805, 49.22920708060482, 0.22412994807665337, 3296873.9711169004, 49.20542650869242, 0.22696895305200793, 3340465.728419431, 49.20926554507314, 0.22972897367720113, 3384633.8624113193, 49.18000182812329, 0.23256085984357344, 3429385.994030769, 49.175626063408984, 0.23618146816643407, 3474729.844981134, 49.16073772867489, 0.23925630894758276, 3520673.239063306, 49.16492500626527, 0.24232568112905134, 3567224.103525603, 49.13571894851171, 0.2453402091596744, 3614390.4704316286, 49.119218875495086, 0.2488133681250619, 3662180.4780460945, 49.11410555269845, 0.25193538461963205, 3710602.3722390863, 49.09376591932315, 0.25560766403372615, 3759664.5079087787, 49.0773692209156, 0.2588535917106808, 3809375.3504230822, 49.05664894894555, 0.26211829792268354, 3859743.477080227, 49.06583612275906, 0.26572228262735914, 3910777.5785887865, 49.045361471004426, 0.26889195660072823, 3962486.4605671414, 49.01375195335831, 0.2729727542726257, 4014879.045062899, 48.988430242747675, 0.2758924893754386, 4067964.372092273, 48.966642062524514, 0.2798624757809066, 4121751.601199946, 48.95216315039579, 0.2836373335255535, 4176250.0130394283, 48.949678795662464, 0.28692203974892944, 4231469.010974442, 48.933927093256045, 0.291131342621884, 4287418.122701349, 48.900871986909294, 0.2949379451488487, 4344107.001893158, 48.853992242308045, 0.2989356306286485, 4401545.429865147, 48.85485621342438, 0.3027403397732656, 4459743.317262627, 48.83688963704516, 0.3066285945977457, 4518710.7057709005, 48.812867754755985, 0.31049141243327844, 4578457.76984796, 48.8159662230358, 0.3147980620751897, 4638994.818479957, 48.760521757079985, 0.31928031562198816, 4700332.296960024, 48.73261114437523, 0.32329179468624386, 4762480.788690475, 48.70325289183386, 0.3276000786585261, 4825451.017008977, 48.68412222231968, 0.33223032164385563, 4889253.847038725, 48.639362219937965, 0.3367464693910624, 4953900.287563224, 48.64865012214332, 0.34088760619382596, 5019401.492925709, 48.58597753369992, 0.3445537687570487, 5085768.76495384, 48.578471860076064, 0.34988830989841063, 5153013.554909677, 48.545982093731226, 0.35439844579195734, 5221147.465465614, 48.511956289446275, 0.3590358244866957, 5290182.252706256, 48.458943255023, 0.36405727126647003, 5360129.828156949, 48.44072374974745, 0.3686516060001556, 5431002.260838954, 48.411697485685096, 0.373391883679427, 5502811.779351966, 48.388453489081655, 0.37847404551297736, 5575570.773983998, 48.372105055029515, 0.383320856474204, 5649291.798849336, 48.34196023552555, 0.38839459885772887, 5723987.574054583, 48.267350062032925, 0.39308848865434737, 5799670.987893529, 48.23063674917057, 0.39901305267595144, 5876355.09907085, 48.19040055521977, 0.4039093084724431, 5954053.138955403, 48.15092937679266, 0.4097337359692983, 6032778.51386312, 48.11048553632329, 0.41494675119437635, 6112544.8073702855, 48.079454895249256, 0.4202950419290804, 6193365.782657193, 48.044054451552945, 0.42566606701372656, 6275255.384883003, 47.96752389875109, 0.4317864217999036, 6358227.743591791, 47.92877805900226, 0.4371301677033375, 6442297.175150612, 47.859163606007655, 0.44327495899810776, 6527478.185219603, 47.83554866058043, 0.44903489771207605, 6613785.471254943, 47.78897571860035, 0.45472581143766716, 6701233.925044711, 47.713169470982805, 0.4607817398438603, 6789838.63527847, 47.684029447357005, 0.46712836880341657, 6879614.890150623, 47.60212131108836, 0.4731899329932316, 6970578.179998407, 47.54536518360162, 0.4795568381229129, 7062744.1999745425, 47.495769995364064, 0.48578892242028915, 7156128.852755445, 47.44638282456419, 0.4923972079232773, 7250748.251285023, 47.3570732827636, 0.4990343485480671, 7346618.7215549825, 47.29418229689904, 0.5052840942897808, 7443756.80542167, 47.24155034813156, 0.5123014208647428, 7542179.263460315, 47.18232027311458, 0.5188038180777349, 7641903.077857005, 47.151855110149484, 0.5260821169529987, 7742945.455338757, 47.039424894704396, 0.532522029695437, 7845323.830142545, 46.97316329339159, 0.5398324299274463, 7949055.867023354, 46.884878636922004, 0.5474686200746333, 8054159.464302249, 46.80994496572298, 0.5545494905122645, 8160652.756954485, 46.72708862334453, 0.5617800173137281, 8268554.11973872, 46.65313950006084, 0.5692004825707987, 8377882.170367336, 46.621672098385815, 0.5768478784859603, 8488655.772718938, 46.495384289512074, 0.5846519960594585, 8600894.04009307, 46.38469462439145, 0.5931262496158722, 8714616.338508228, 46.31327740538186, 0.6001140025549069, 8829842.290043209, 46.20825491028732, 0.6086394178766533, 8946591.776222927, 46.14148354213476, 0.6162865856692903, 9064884.941448696, 46.02617720990913, 0.6251060236283297, 9184742.196474167, 45.90825227993389, 0.6334805384029172, 9306184.221926937, 45.82644538290632, 0.6418752902555024, 9429231.971877005, 45.70584251857653, 0.6501564605082537, 9553906.677452119, 45.60773786361272, 0.6593467904190532, 9680229.850501234, 45.465572242960526, 0.667813483704979, 9808223.287306082, 45.370782547862106, 0.6767479295729664, 9937909.07234215, 45.278286181235394, 0.685787131219018, 10069309.582089063, 45.14831384161517, 0.6953121568621612, 10202447.488891661, 44.99997987228786, 0.7044822142254462, 10337345.764871813, 44.88089893742221, 0.7139720330619045, 10474027.685892282, 44.76294198573418, 0.7243520365025389, 10612516.835572654, 44.61589116502605, 0.7336983990608337, 10752837.109358728, 44.496439232039236, 0.7431494669940389, 10895012.718645347, 44.28757879517352, 0.7528099489018971, 11039068.1949541, 44.18225162666157, 0.7634079763124275, 11185028.394165907, 44.042753956138185, 0.77362300347845, 11332918.500809934, 43.8875226485851, 0.7842045751983888, 11482764.032408835, 43.73822754596332, 0.7959273882926557, 11634590.843881832, 43.54320014305958, 0.8062734327585716, 11788425.132005634, 43.37053461263363, 0.8180980302803776, 11944293.439934723, 43.16912139490801, 0.8291073121875452, 12102222.661781007, 43.04915831580196, 0.8396431029781101, 12262240.047254441, 42.89142259952636, 0.8516296644183309, 12424373.20636459, 42.67733932056135, 0.863326037794432, 12588650.114184767, 42.41171107091929, 0.875185930983658, 12755099.115678756, 42.23531710571934, 0.8872120203875512, 12923748.930591768, 42.056258192411306, 0.8997626950473533, 13094628.658405645, 41.83519120310027, 0.9123586560713152, 13267767.783360004, 41.6370311074584, 0.9246314722769271, 13443196.17953935, 41.387745330690066, 0.9378924941839707, 13620944.116027886, 41.23447242930132, 0.9506855680241261, 13801042.262132019, 40.96358906298593, 0.9644505152101008, 13983521.692672404, 40.699126440376645, 0.9776153294055029, 14168413.89334547, 40.43982787937423, 0.9917259680078826, 14355750.766156318, 40.23182779001589, 1.0055063560338355, 14545564.63492298, 39.961443440605, 1.0196058937392316, 14737888.250853932, 39.67372326288413, 1.0335476240162398, 14932754.798198868, 39.44243296257215, 1.0488045514072986, 15130197.899974689, 39.14518044974827, 1.0638725921277299, 15330251.623766689, 38.84200832811587, 1.0795046665916752, 15532950.487606961, 38.57516098790695, 1.0959691905147895, 15738329.465930022, 38.22574608407651, 1.11085629775608, 15946423.995607682, 37.96866733286538, 1.1274793940802126, 16157269.982063202, 37.61206259587007, 1.1429396862841243, 16370903.805466818, 37.28356321837679, 1.1610625674795811, 16587362.327012643, 36.96079578230925, 1.1770711339673687, 16806682.89527911, 36.656886880661304, 1.1945275878710337, 17028903.35267296, 36.24005948106828, 1.212702879740254, 17254062.04195901, 35.909335288572485, 1.2310786735469534, 17482197.81287565, 35.55025009309201, 1.2499055596998956, 17713350.02883844, 35.146970940166455, 1.2681880317681598, 17947558.57373171, 34.77824051289354, 1.288226884002255, 18184863.85879058, 34.35446234361975, 1.3081334159140878, 18425306.82957338, 33.94943584106224, 1.3275225587561483, 18668928.973026842, 33.53759222248398, 1.3495562331816007, 18915772.324644115, 33.09751895836192, 1.3707828173860923, 19165879.475718036, 32.68384138287976, 1.3926802344198241, 19419293.580689687, 32.229916286229525, 1.413527291240001, 19676058.36459474, 31.724811642856494, 1.4370666792071265, 19936218.130607612, 31.272227225267624, 1.461734940538952, 20199817.76768605, 30.77483805846476, 1.4853142332969613, 20466902.75831609, 30.34583883680933, 1.5106814986513, 20737519.186360124, 29.78259126354139, 1.5360156615102387, 21011713.745008055, 29.26857690291324, 1.5622393864358861, 21289533.744834237, 28.71798279155055, 1.5895388321433046, 21571027.121960297, 28.201980064577462, 1.617870026368402, 21856242.44632656, 27.643209613771408, 1.6470745694248854, 22145228.93007214, 27.061208013167267, 1.6774269900775038, 22438036.43602653, 26.482162071178973, 1.708201908956807, 22734715.48631279, 25.879119492460774, 1.7422551555109946, 23035317.27106518, 25.32704553599189, 1.7743086312608813, 23339893.65726132, 24.718764131960306, 1.8104192587444214, 23648497.197671916, 24.032465898223524, 1.8474327732445142, 23961181.13992801, 23.405535837112208, 1.8850339440641406, 24277999.435708925, 22.78041277255093, 1.9257533176575783, 24599006.75005091, 22.158347788164175, 1.9675118655261614, 24924258.470779642, 21.453518815624506, 2.011807513224275, 25253810.718066644, 20.771389678726933, 2.0585418384959047, 25587720.354112897, 20.12200046611648, 2.1089498142713956, 25926044.992959637, 19.396077355348233, 2.162608986377453, 26268843.010429718, 18.822324318409134, 2.2163951143146248, 26616173.554199588, 18.083649443964216, 2.2767711191210305, 26968096.55400526, 17.455510954849345, 2.3413071387170103, 27324672.731982414, 16.791769777597583, 2.411593629272314, 27685963.61314404, 16.15663825364541, 2.481615162139117, 28052031.535995767, 15.59938536803191, 2.5635275186778586, 28422939.663292423, 15.013215966470083, 2.6484610151548864, 28798751.992935944, 14.45515452465021, 2.741755060179058, 29179533.369018253, 14.027092950113936, 2.8434225407598217, 29565349.493009254, 13.65748035027174, 2.9482677296109197, 29956266.935093682, 13.40635497213106, 3.066526725089525, 30352353.14565691, 13.137593644047852, -3.099571409150509, 30753676.466923553, 13.070489942067788, -2.975306143106237, 31160306.14474903, 13.11859382207868, -2.845287051442727, 31572312.340568002, 13.275464805350099, -2.7152111666720256, 31989766.143499773, 13.619525836228181, -2.5885359103364043, 32412739.58261481, 14.10562371164106, -2.465902112489834, 32841305.639362372, 14.687206067162032, -2.3415630230444133, 33275538.26016356, 15.449607664949696, -2.2289692324373402, 33715512.369169764, 16.327590047188114, -2.1189301602567636, 34161303.881190896, 17.350856316293264, -2.0144577973778275, 34612989.714793496, 18.40949910485038, -1.922269357159236, 35070647.80557308, 19.64699190509497, -1.830892390356288, 35534357.119600914, 20.95538337515062, -1.7468587061215894, 36004197.66704966, 22.367320953922004, -1.670097893030782, 36480250.515998095, 23.828547317075113, -1.5997119954606223, 36962597.80641944, 25.373171730304986, -1.5273967754583382, 37451322.76435357, 27.01616945465279, -1.4633901599646038, 37946509.71626771, 28.727976623988656, -1.4009637831326451, 38448244.10360586, 30.574854240120846, -1.3394892983184998, 38956612.49753177, 32.46035974677084, -1.2843616594395901, 39471702.61386569, 34.295489947603826, -1.2308293538098096, 39993603.32821977, 36.301402020261676, -1.1768241268779192, 40522404.6913324, 38.32740213081458, -1.127448480210949, 41058197.94460653, 40.45367445118702, -1.0768088562412859, 41601075.53585213, 42.58733947527955, -1.028832767749417, 42151131.13523822, 44.808625791285316, -0.9811222761528726, 42708459.65145435, 47.08216258948301, -0.935112157289252, 43273157.248087205, 49.434790293495666, -0.8875533077860994, 43845321.36021234, 51.76770611411167, -0.8431972152684872, 44425050.71120671, 54.277218616016064, -0.7966568673254142, 45012445.32978207, 56.78753163037345, -0.7517834881701105, 45607606.567245014, 59.31659165629515, -0.7074098013436436, 46210637.11498379, 61.96364962420367, -0.664662012670831, 46821641.02218782, 64.55230974309742, -0.6175162469209541, 47440723.713799976, 67.42021013911388, -0.5738928477590169, 48067992.00870777, 70.21989683820456, -0.5299800629351139, 48703554.13817351, 73.09080745040224, -0.4822581496763467, 49347519.76450975, 76.21550623989967, -0.43759636993289514, 49999999.99999999, 79.14205777660682, -0.3930038086422039]}, ...(3 in all)]
  in  "R (Ohms)":dbl format="%#_6p"
  out "Calibration R (Ohm)":T4(graph)
  in  "Type":i16(ring)=2 items=["R || C"=2]
  in  "Ref 2":dbl caption="C (F)" format="%#_6p"
  in  "Ref 3":dbl format="%#_6p"
  out "ziCalib":T6
  in  "stop":bool
  in  "Averaging":u16(ring)=1 items=["1"=1, "2"=2, "4"=4, "16"=16, "32"=32, "64"=64]
  in  "Bandwidth (Hz)":dbl=-1.0 format="%#_p"
  in  "Precision":u16(ring) items=["Low", "Med", "High"]
  in  "Number of Points":i32=100 caption="Points" min=2 max=66000
  in  "Filter Order":i32(ring)=4 items=["6, 1st"=1, "12, 2nd"=2, "18, 3rd"=3, "24, 4th"=4, "30, 5th"=5, "36, 6th"=6, "42, 7th"=7, "48, 8th"=8]
  in  "Stop (Hz)":dbl=1000000.0 format="%_5p"
  in  "Start (Hz)":dbl=10000.0 format="%_5p"
  # "Tested Devices:\n- HF2IS\nNot supported:\n- UHFLI"
  # "Requires HF2IS or HF2LI-MF and assumes \noscillator 1 on signal output 1 for stimulation"
  # "Actual Reading"
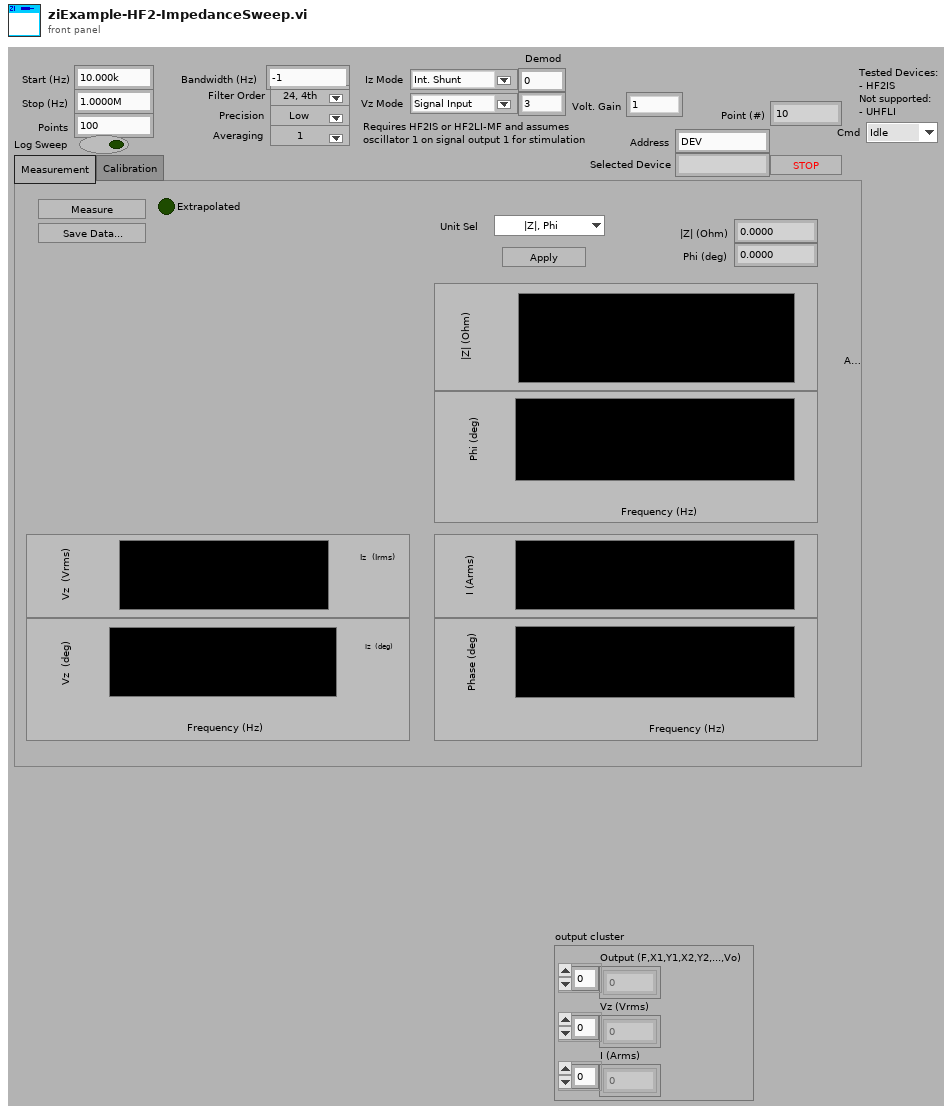
[diagram p1: front panel]
types:
  T1 = cluster{"Output (F,X1,Y1,X2,Y2,...,Vo)":dbl[], "Vz (Vrms)":cdb[], "I (Arms)":cdb[]}
  T2 = cluster{"Output (F,X1,Y1,X2,Y2,...,Vo)":dbl[], dbl[]}[]
  T3 = typedef "Zurich Instruments LabOne.lvlib/ziTypeImpedanceEqCircModel.ctl" = enum16{"Invalid", "|Z|, Phi", "R||C", "R||L", "R*C", "D*C", "R*L", "ReZ, ImZ", "G, B"}
  T4 = cluster{"Output (F,X1,Y1,X2,Y2,...,Vo)":dbl[], dbl[]}
  T5 = cluster{"Ref Label":string, "Ref ID":i16, "Ref_Z":cdb[], "Meas_Z":dbl[][]}[]
  T6 = typedef "Zurich Instruments LabOne.lvlib/ziTypeCalib.ctl" = cluster{"Time Stamp":timestamp, "Calib Model":T7, "ModelCoeffs":cdb[], "Meas (F,Z0,...,Zn)":dbl[][]}
  T7 = typedef "Zurich Instruments LabOne.lvlib/ziTypeCalibModel.ctl" = enum16{"Invalid", "Unity", "R||C", "R||L", "R*C", "R*L"}
  T8 = typedef "Zurich Instruments LabOne.lvlib/ziTypeHandle.ctl" = cluster{"handleValid":bool, "Conn":u64, "Path Prefix":string, "Handle":u64, "Connected":bool, "Clockbase(s)":dbl}
  T9 = enum16{"big-endian, network order", "native, host order", "little-endian"}
  T10 = cluster{"Output (F,X1,Y1,X2,Y2,...,Vo)":dbl[], "Values":dbl[]}
  T11 = typedef "LVRangeTypeDef.ctl" = cluster{"Minimum":dbl, "Maximum":dbl, "Increment":dbl, "Minor Increment":dbl, "Start":dbl}
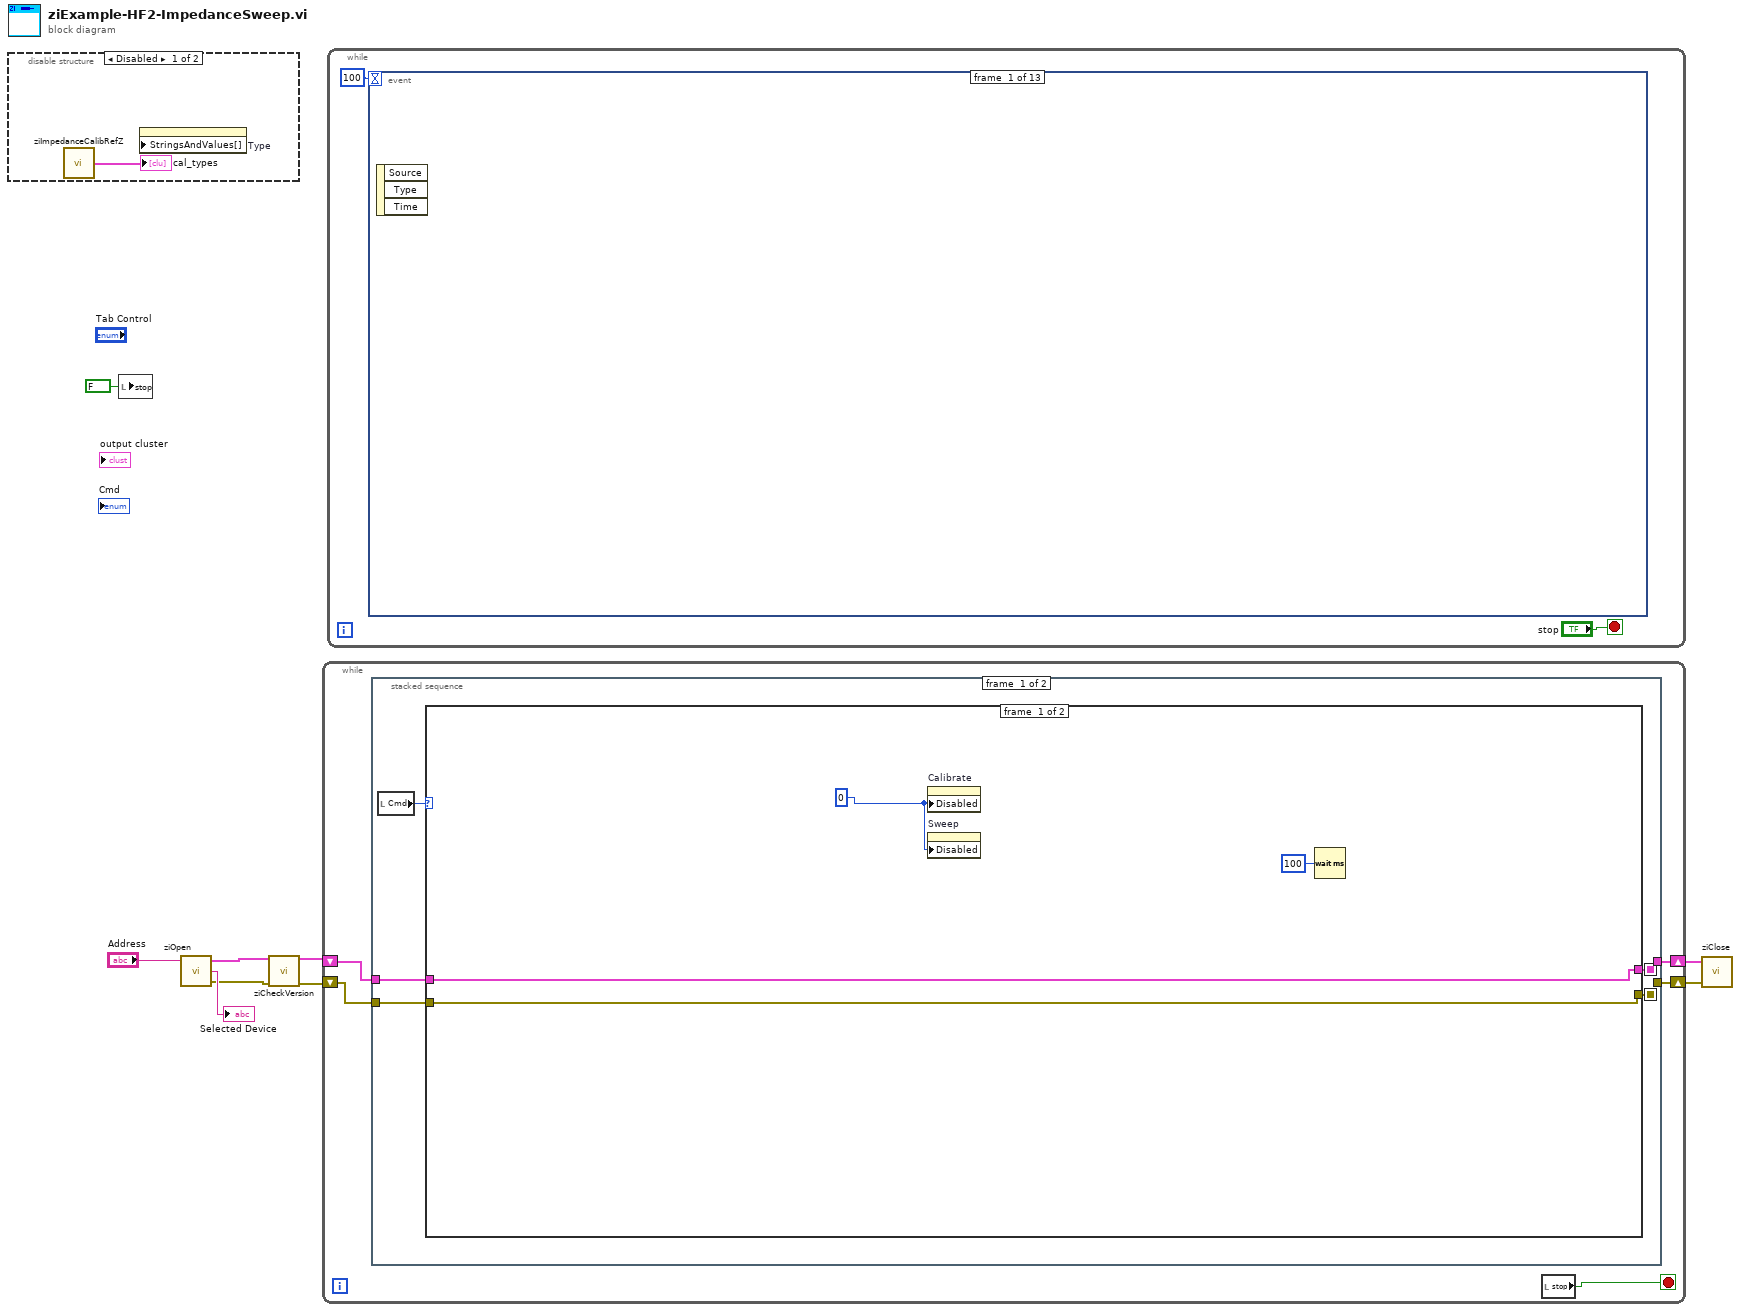
[diagram p0: block diagram]
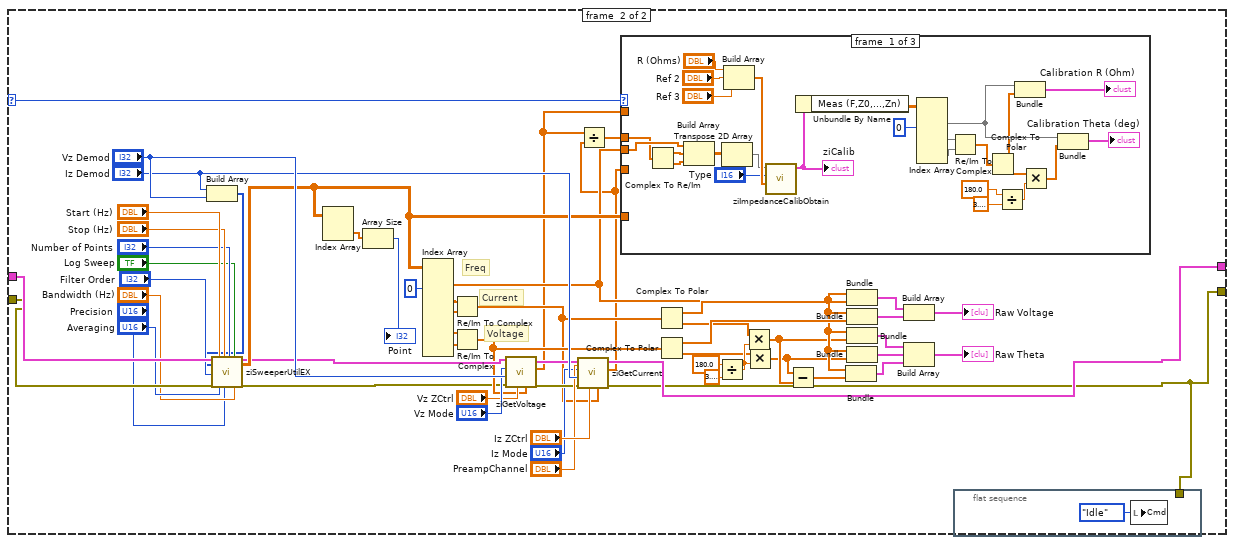
[diagram p2: hidden frame]
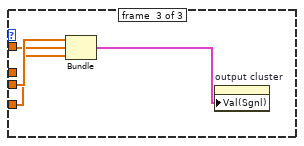
[diagram p4: hidden frame]
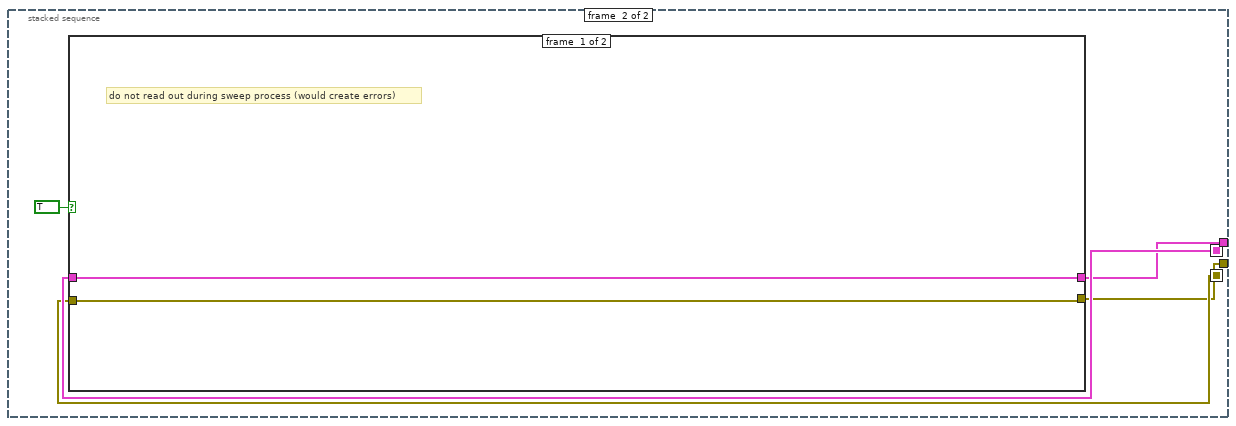
[diagram p5: hidden frame]
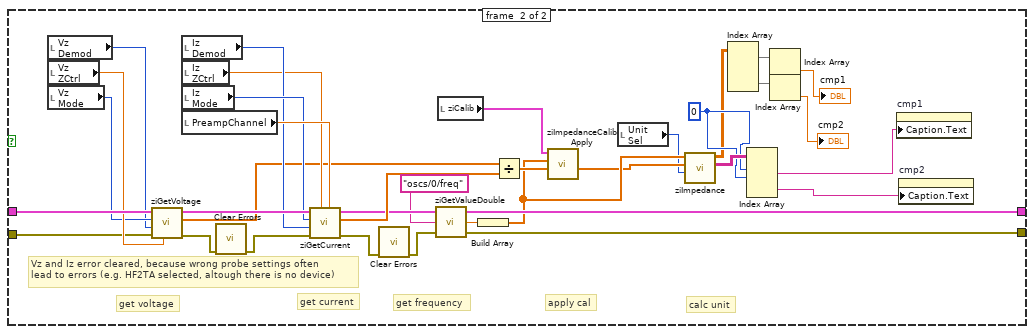
[diagram p6: hidden frame]
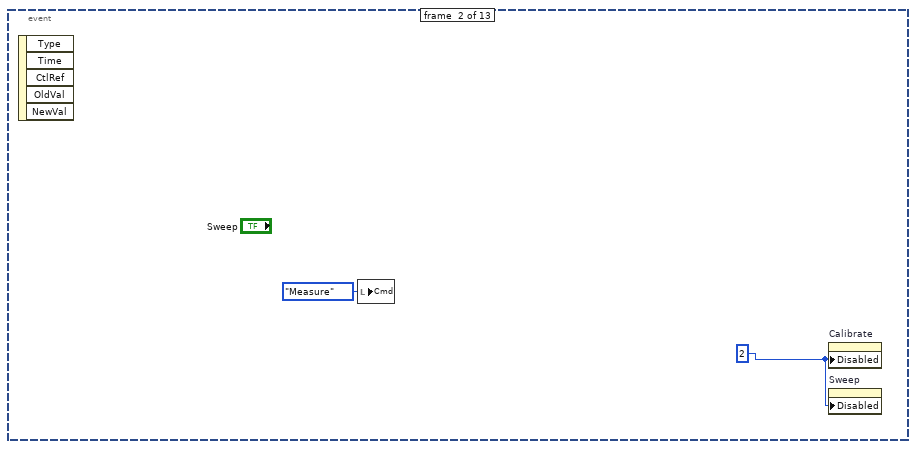
[diagram p8: hidden frame]
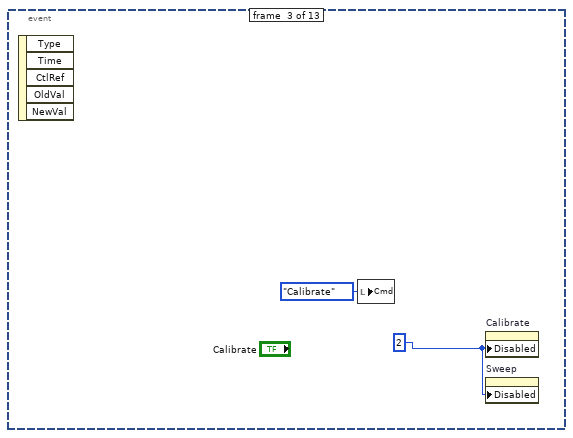
[diagram p9: hidden frame]
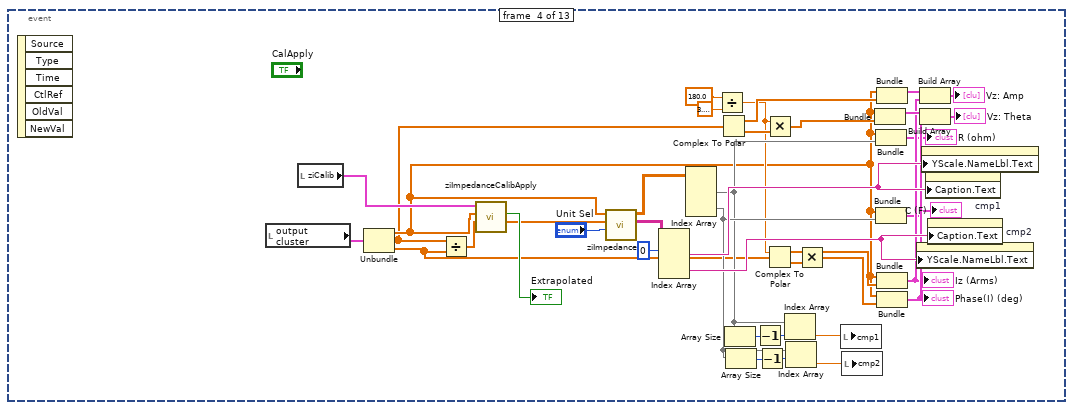
[diagram p10: hidden frame]
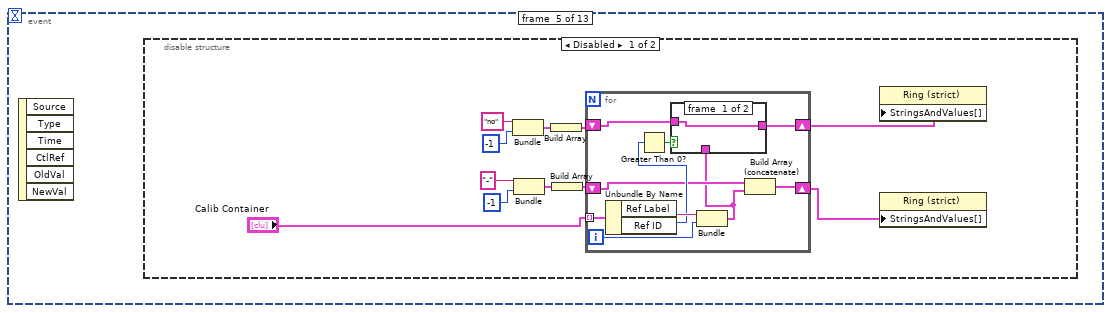
[diagram p11: hidden frame]
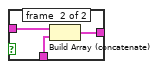
[diagram p12: hidden frame]
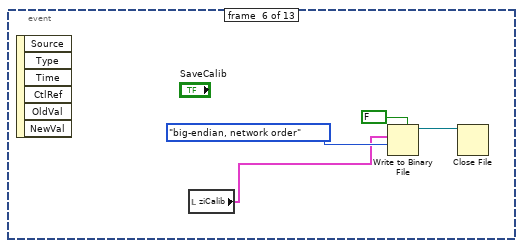
[diagram p14: hidden frame]
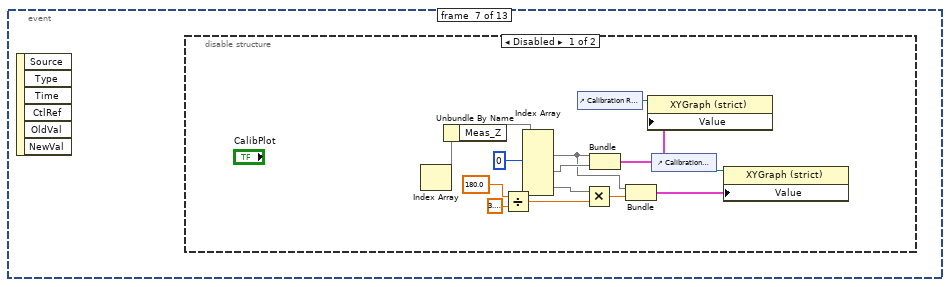
[diagram p15: hidden frame]
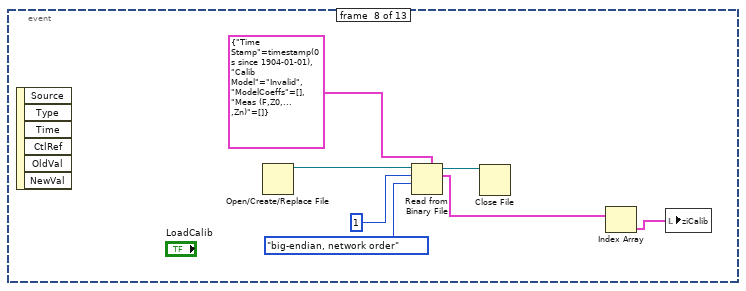
[diagram p17: hidden frame]
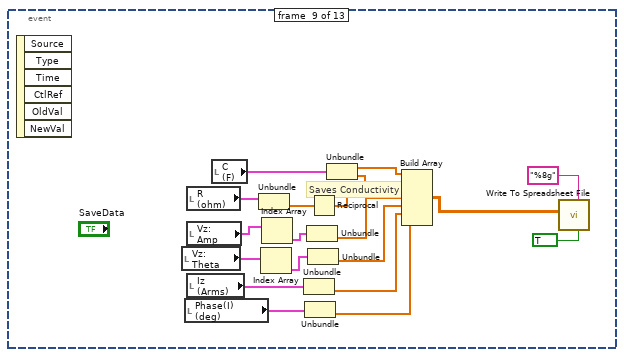
[diagram p18: hidden frame]
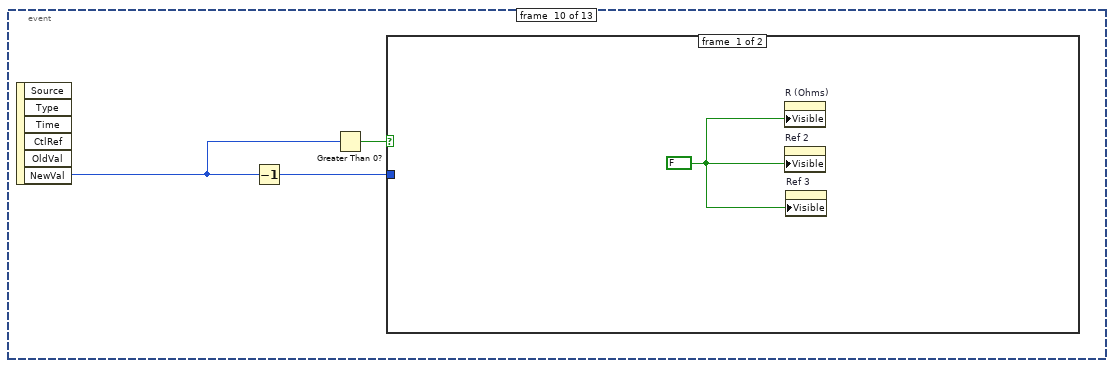
[diagram p19: hidden frame]
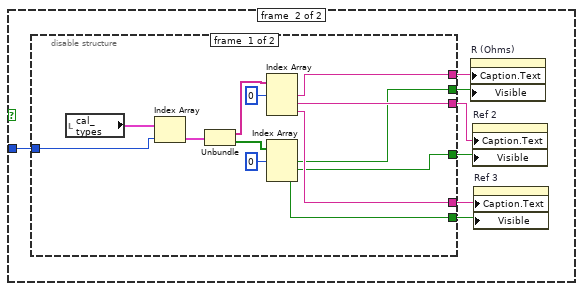
[diagram p20: hidden frame]
diagram:
  n1 = disable-structure shown="Disabled" {
    frame #0 {
      n2 = call <instrlib>:"ziImpedanceCalibRefZ.vi"() -> ("cal_types"=→"cal_types":cluster{string[], bool[]}[])  [unwired: 4 in, 1 out]
      n3 = property on="Type" class="Ring (strict)" props=["StringsAndValues[]"]() -> ()  [unwired: 3 in, 2 out]
    }
    frame #1 {
    }
  }
  n4 = local write "stop"(FALSE ("stop")) -> ()
  n5 = call <instrlib>:"ziOpen.vi"("Address"="Address") -> ("Error Out"=w1:errorcluster, "Selected Device"=→"Selected Device":string, "HandleOut"=w2:T8)  [unwired: 3 in]
  n6 = call <instrlib>:"ziCheckVersion.vi"("Handle In"=w2, "Error In"=w1) -> ("Handle Out"=w4:T8, "Error Out"=w3:errorcluster)  [unwired: 11 in, 1 out]
  n7 = while {
    shift-right: [w12] -> w9
    shift-left: w4 -> [w14]
    shift-right: [w11] -> w8
    shift-left: w3 -> [w13]
    stop <- w15 stop-if-true
    n8 = stacked-sequence {
      seq-local: [w17 _] -> [_ w115]
      seq-local: [w16 _] -> [_ w114]
      tunnel: w14 -> [w20 _]
      tunnel: w13 -> [w19 _]
      tunnel: [_ w113] -> w12
      tunnel: [_ w112] -> w11
      frame #0 {
        n9 = local read "Cmd"() -> (w18:enum16{"Idle", "Calibrate", "Measure"})
        n10 = case shown="\"Calibrate\", \"Measure\"" w18 {
          selector: w18 -> [_ w78]
          tunnel: w20 -> [w23 w74]
          tunnel: w19 -> [w22 w35]
          tunnel: [w23 w77] -> w17
          tunnel: [w22 w76] -> w16
          frame #0 {
            w24 = u8 0 ("Disabled")
            n11 = property on="Calibrate" class="Bool"("Disabled"=w24) -> ()  [unwired: 2 in, 2 out]
            n12 = property on="Sweep" class="Bool"("Disabled"=w24) -> ()  [unwired: 2 in, 2 out]
            n13 = Wait (ms)(milliseconds to wait=u32 100) -> ()  [unwired: 1 out]
          }
          frame #1 {
            # "Voltage"
            # "Current"
            # "Freq"
            n14 = Build Array("Iz Demod", "Vz Demod") -> (w26:i32[])
            n15 = call <instrlib>:"ziSweeperUtilEX.vi"("Handle In"=w74, "Input Demods (0)"=w26, "Order (4)"="Filter Order", "Error In"=w35, "Start (Hz)"="Start (Hz)", "average"="Averaging", "Stop (Hz)"="Stop (Hz)", "Precision (Low)"="Precision", "Steps (#)"="Number of Points", "Log Sweep (true)"="Log Sweep", "Bandwith (-1=auto)"="Bandwidth (Hz)") -> ("Handle Out"=w73:T8, "Output (F,X1,Y1,X2,Y2,...,Vo)"=w75:dbl[][], "Error Out"=w34:errorcluster)  [unwired: 6 in]
            n16 = Index Array(array=w75) -> (element=w37:dbl[])  [unwired: 2 in]
            n17 = Array Size(array=w37) -> (size(s)=→"Point":i32)
            n18 = Index Array(array=w75, index (col) #1=0 ("index (row)")) -> (element #1=w56:dbl[], element #2=w59:dbl[], element #3=w60:dbl[], element #4=w58:dbl[], element #5=w54:dbl[])  [unwired: 9 in]
            n19 = Re/Im To Complex(1:w60, 2:w59) -> (0:w41:cdb[])
            n20 = Re/Im To Complex(1:w54, 2:w58) -> (0:w42:cdb[])
            n21 = call <instrlib>:"ziGetVoltage.vi"("DemodVoltage (Vrms)"=w42, "ZCtrl / Gain (0)"="Vz ZCtrl", "error in"=w34, "Demodulator (0)"="Vz Demod", "Mode"="Vz Mode", "handle in"=w73) -> ("error out"=w50:errorcluster, "Vz (Vrms)"=w40:cdb[], "handle out"=w49:T8)  [unwired: 3 in]
            n22 = call <instrlib>:"ziGetCurrent.vi"("Opt: DemodVoltage (Vrms)"=w41, "PreampCh / Gain(0)"="PreampChannel", "ZCtrl / Shunt (0)"="Iz ZCtrl", "Error in"=w50, "Demodulator (0)"="Iz Demod", "Mode"="Iz Mode", "Handle in"=w49) -> ("Error out"=w76:errorcluster, "I (Arms)"=w39:cdb[], "Handle out"=w77:T8)  [unwired: 2 in]
            n23 = Divide(x=w40, y=w39) -> (x/y=w38:cdb[])
            n24 = case shown="\"Measure\"" w78 {
              tunnel: w56 -> [w87 _ w110]
              tunnel: w40 -> [_ _ w109]
              tunnel: w39 -> [_ _ w108]
              tunnel: w75 -> [_ _ _]
              tunnel: w38 -> [w82 _ _]
              frame #0 {
                n25 = Complex To Re/Im(x + iy=w82) -> (x=w86:dbl[], y=w85:dbl[])
                n26 = Build Array(w87, w86, w85) -> (w84:dbl[][])
                n27 = Transpose 2D Array(2D array=w84) -> (transposed array=w83:dbl[][])
                n28 = Build Array("R (Ohms)", "Ref 2", "Ref 3") -> (w93:dbl[])
                n29 = call <instrlib>:"ziImpedanceCalibObtain.vi"("Ref_Z"=w93, "Ref ID"="Type", "Measurement (F,Z0,..,Zn)"=w83) -> ("ziCalib"=w94:T6)  [unwired: 5 in]
                "ziCalib" <- w94
                n30 = Unbundle By Name(w94) -> ("Meas (F,Z0,...,Zn)"=w104:dbl[][])
                n31 = Index Array(array=w104, index (col) #1=0 ("index (row)")) -> (element #1=w103:dbl[], element #2=w91:dbl[], element #3=w90:dbl[])  [unwired: 5 in]
                n32 = Re/Im To Complex(1:w90, 2:w91) -> (0:w81:cdb[])
                n33 = Complex To Polar(r * e^(i*theta)=w81) -> (r=w88:dbl[], theta=w89:dbl[])
                n34 = Divide(x=180.0, y=3.141592653589793) -> (x/y=w97:dbl)
                n35 = Bundle("Meas (F,Z0,...,Zn)"=w103, w88) -> (→"Calibration R (Ohm)":cluster{"Meas (F,Z0,...,Zn)":dbl[], dbl[]})  [unwired: 1 in]
                n36 = Multiply(x=w89, y=w97) -> (x*y=w98:dbl[])
                n37 = Bundle("Meas (F,Z0,...,Zn)"=w103, w98) -> (→"Calibration Theta (deg)":cluster{"Meas (F,Z0,...,Zn)":dbl[], dbl[]})  [unwired: 1 in]
              }
              frame #1 {
              }
              frame #2 {
                n38 = Bundle("Output (F,X1,Y1,X2,Y2,...,Vo)"=w110, "Vz (Vrms)"=w109, "I (Arms)"=w108) -> (w107:T1)  [unwired: 1 out]
                n39 = property on="output cluster" class="Clust (strict)"("Val(Sgnl)"=w107) -> ()  [unwired: 2 in, 2 out]
              }
            }
            n40 = Complex To Polar(r * e^(i*theta)=w41) -> (r=w66:dbl[], theta=w53:dbl[])
            n41 = Complex To Polar(r * e^(i*theta)=w42) -> (r=w65:dbl[], theta=w61:dbl[])
            n42 = Divide(x=180.0, y=3.141592653589793) -> (x/y=w62:dbl)
            n43 = Multiply(x=w53, y=w62) -> (x*y=w46:dbl[])
            n44 = Multiply(x=w61, y=w62) -> (x*y=w45:dbl[])
            n45 = Subtract(x=w45, y=w46) -> (x-y=w47:dbl[])
            n46 = Bundle("Output (F,X1,Y1,X2,Y2,...,Vo)"=w56, w47) -> (w67:T4)  [unwired: 1 out]
            n47 = Bundle("Output (F,X1,Y1,X2,Y2,...,Vo)"=w56, w66) -> (w55:T4)  [unwired: 1 out]
            n48 = Bundle("Output (F,X1,Y1,X2,Y2,...,Vo)"=w56, w65) -> (w72:T4)  [unwired: 1 out]
            n49 = Bundle("Output (F,X1,Y1,X2,Y2,...,Vo)"=w56, w46) -> (w68:T4)  [unwired: 1 out]
            n50 = Bundle("Output (F,X1,Y1,X2,Y2,...,Vo)"=w56, w45) -> (w69:T4)  [unwired: 1 out]
            n51 = Build Array(w55, w72) -> (→"Raw Voltage":T2)
            n52 = Build Array(w68, w69, w67) -> (→"Raw Theta":T2)
            n53 = flat-sequence {
              tunnel: w76 -> [_]
              frame #0 {
                n54 = local write "Cmd"(enum16{"Idle", "Calibrate", "Measure"}."Idle" ("Cmd")) -> ()
              }
            }
          }
        }
      }
      frame #1 {
        n55 = case shown="True" TRUE {
          tunnel: w115 -> [w118 w153]
          tunnel: [w118 w139] -> w113
          tunnel: [w117 w138] -> w112
          tunnel: w114 -> [w117 w134]
          frame #0 {
            # "do not read out during sweep process (would create errors)"
          }
          frame #1 {
            w124 = 0 ("disabled index (col)")
            # "Vz and Iz error cleared, because wrong probe settings often \nlead to errors (e.g. HF2TA selected, altough there is no device)"
            # "calc unit"
            # "apply cal"
            # "get frequency"
            # "get current"
            # "get voltage"
            n56 = local read "Vz Demod"() -> (w150:i32)
            n57 = local read "Vz ZCtrl"() -> (w152:dbl)
            n58 = local read "Vz Mode"() -> (w151:u16)
            n59 = call <instrlib>:"ziGetVoltage.vi"("ZCtrl / Gain (0)"=w152, "error in"=w134, "Demodulator (0)"=w150, "Mode"=w151, "handle in"=w153) -> ("error out"=w133:errorcluster, "Vz (Vrms)"=w144:cdb[], "handle out"=w149:T8)  [unwired: 4 in]
            n60 = local read "Iz Demod"() -> (w146:i32)
            n61 = local read "Iz ZCtrl"() -> (w145:dbl)
            n62 = local read "Iz Mode"() -> (w147:u16)
            n63 = local read "PreampChannel"() -> (w148:dbl)
            n64 = call <vilib>:"Clear Errors.vi"("error in (no error)"=w133) -> ("error out"=w132:errorcluster)  [unwired: 6 in]
            n65 = call <instrlib>:"ziGetCurrent.vi"("PreampCh / Gain(0)"=w148, "ZCtrl / Shunt (0)"=w145, "Error in"=w132, "Demodulator (0)"=w146, "Mode"=w147, "Handle in"=w149) -> ("Error out"=w131:errorcluster, "I (Arms)"=w143:cdb[], "Handle out"=w141:T8)  [unwired: 3 in]
            n66 = call <vilib>:"Clear Errors.vi"("error in (no error)"=w131) -> ("error out"=w130:errorcluster)  [unwired: 6 in]
            n67 = call <instrlib>:"ziGetValueDouble.vi"("error in"=w130, "Path"="oscs/0/freq", "Handle in"=w141) -> ("error out"=w138:errorcluster, "Value"=w137:dbl, "Handle out"=w139:T8)
            n68 = local read "ziCalib"() -> (w129:T6)
            n69 = Build Array(w137) -> (w136:dbl[])
            n70 = Divide(x=w144, y=w143) -> (x/y=w142:cdb[])
            n71 = call <instrlib>:"ziImpedanceCalibApply.vi"("Measurement"=w142, "Frequencies (Hz)"=w136, "ziCalib In"=w129) -> ("Corrected Measurement"=w135:cdb[])  [unwired: 4 in, 2 out]
            n72 = local read "Unit Sel"() -> (w128:T3)
            n73 = call <instrlib>:"ziImpedance.vi"("Eq Model"=w128, "Z (Ohm)"=w135, "Frequency (Hz)"=w136) -> ("Labels and Units"=w127:string[][], "Values"=w122:dbl[][])  [unwired: 7 in]
            n74 = Index Array(array=w122) -> (element #1=w121:dbl[], element #2=w120:dbl[])  [unwired: 4 in]
            n75 = Index Array(array=w127, index (row) #1=w124, index (col) #1=w124) -> (element #1=w126:string, element #2=w125:string)  [unwired: 2 in]
            n76 = Index Array(array=w121) -> (element=→"cmp1":dbl)  [unwired: 1 in]
            n77 = Index Array(array=w120) -> (element=→"cmp2":dbl)  [unwired: 1 in]
            n78 = property on="cmp1" class="DigNum (strict)"("Caption.Text"=w126) -> ()  [unwired: 2 in, 2 out]
            n79 = property on="cmp2" class="DigNum (strict)"("Caption.Text"=w125) -> ()  [unwired: 2 in, 2 out]
          }
        }
      }
    }
    n80 = local read "stop"() -> (w15:bool)
  }
  n81 = while {
    stop <- "stop" stop-if-true
    n82 = event shown="[5] \"SaveCalib\": Value Change" {
      selector: _ -> [_ _ _ _ _ _ _ _ _ _ _ _ _]
      dyn-events: _ -> [_ _ _ _ _ _ _ _ _ _ _ _ _]
      timeout: 100 -> [_ _ _ _ _ _ _ _ _ _ _ _ _]
      event #0 {
        n83 = event-data() -> ()  [unwired: 1 in, 3 out]
      }
      event #1 {
        w156 = u8 2 ("Disabled")
        n84 = event-data() -> ()  [unwired: 1 in, 5 out]
        n85 = local write "Cmd"(enum16{"Idle", "Calibrate", "Measure"}."Measure" ("Cmd")) -> ()
        n86 = property on="Calibrate" class="Bool"("Disabled"=w156) -> ()  [unwired: 2 in, 2 out]
        n87 = property on="Sweep" class="Bool"("Disabled"=w156) -> ()  [unwired: 2 in, 2 out]
      }
      event #2 {
        w158 = u8 2 ("Disabled")
        n88 = event-data() -> ()  [unwired: 1 in, 5 out]
        n89 = local write "Cmd"(enum16{"Idle", "Calibrate", "Measure"}."Calibrate" ("Cmd")) -> ()
        n90 = property on="Calibrate" class="Bool"("Disabled"=w158) -> ()  [unwired: 2 in, 2 out]
        n91 = property on="Sweep" class="Bool"("Disabled"=w158) -> ()  [unwired: 2 in, 2 out]
      }
      event #3 {
        w196 = 0 ("index (row)")
        n92 = event-data() -> ()  [unwired: 1 in, 6 out]
        n93 = local read "output cluster"() -> (w170:T1)
        n94 = local read "ziCalib"() -> (w167:T6)
        n95 = Unbundle(w170) -> ("Output (F,X1,Y1,X2,Y2,...,Vo)"=w162:dbl[], "Vz (Vrms)"=w160:cdb[], "I (Arms)"=w161:cdb[])
        n96 = Divide(x=w160, y=w161) -> (x/y=w165:cdb[])
        n97 = call <instrlib>:"ziImpedanceCalibApply.vi"("Measurement"=w165, "Frequencies (Hz)"=w162, "ziCalib In"=w167) -> ("Corrected Measurement"=w166:cdb[], "Extrapolated"=→"Extrapolated":bool)  [unwired: 4 in, 1 out]
        n98 = call <instrlib>:"ziImpedance.vi"("Eq Model"="Unit Sel", "Z (Ohm)"=w166, "Frequency (Hz)"=w162) -> ("Labels and Units"=w163:string[][], "Values"=w164:dbl[][])  [unwired: 7 in]
        n99 = Index Array(array=w163, index (row) #1=w196, index (col) #1=w196) -> (element #1=w197:string, element #2=w198:string)  [unwired: 2 in]
        n100 = Index Array(array=w164) -> (element #1=w194:dbl[], element #2=w195:dbl[])  [unwired: 4 in]
        n101 = Divide(x=180.0, y=3.141592653589793) -> (x/y=w175:dbl)
        n102 = Complex To Polar(r * e^(i*theta)=w160) -> (r=w179:dbl[], theta=w176:dbl[])
        n103 = Array Size(array=w194) -> (size(s)=w188:i32)
        n104 = Array Size(array=w195) -> (size(s)=w191:i32)
        n105 = Decrement(x=w188) -> (x-1=w189:i32)
        n106 = Decrement(x=w191) -> (x-1=w190:i32)
        n107 = Multiply(x=w175, y=w176) -> (x*y=w177:dbl[])
        n108 = Complex To Polar(r * e^(i*theta)=w161) -> (r=w178:dbl[], theta=w174:dbl[])
        n109 = Index Array(array=w194, index=w189) -> (element=w192:dbl)
        n110 = Index Array(array=w195, index=w190) -> (element=w193:dbl)
        n111 = Multiply(x=w175, y=w174) -> (x*y=w181:dbl[])
        n112 = local write "cmp1"(w192) -> ()
        n113 = local write "cmp2"(w193) -> ()
        n114 = Bundle("Output (F,X1,Y1,X2,Y2,...,Vo)"=w162, w177) -> (w185:T4)  [unwired: 1 out]
        n115 = Bundle("Output (F,X1,Y1,X2,Y2,...,Vo)"=w162, "Values"=w194) -> (→"R (ohm)":T10)  [unwired: 1 out]
        n116 = Bundle("Output (F,X1,Y1,X2,Y2,...,Vo)"=w162, "Values"=w195) -> (→"C (F)":T10)  [unwired: 1 out]
        n117 = Bundle("Output (F,X1,Y1,X2,Y2,...,Vo)"=w162, w179) -> (w183:T4)  [unwired: 1 out]
        n118 = Bundle("Output (F,X1,Y1,X2,Y2,...,Vo)"=w162, w178) -> (w184:T4)  [unwired: 1 out]
        "Iz (Arms)" <- w184
        n119 = Bundle("Output (F,X1,Y1,X2,Y2,...,Vo)"=w162, w181) -> (w186:T4)  [unwired: 1 out]
        "Phase(I) (deg)" <- w186
        n120 = property on="C (F)" class="XYGraph (strict)"("YScale.NameLbl.Text"=w198) -> ()  [unwired: 2 in, 2 out]
        n121 = Build Array(w183, w184) -> (→"Vz: Amp":T2)
        n122 = Build Array(w185, w186) -> (→"Vz: Theta":T2)
        n123 = property on="R (ohm)" class="XYGraph (strict)"("YScale.NameLbl.Text"=w197) -> ()  [unwired: 2 in, 2 out]
        n124 = property on="cmp1" class="DigNum (strict)"("Caption.Text"=w197) -> ()  [unwired: 2 in, 2 out]
        n125 = property on="cmp2" class="DigNum (strict)"("Caption.Text"=w198) -> ()  [unwired: 2 in, 2 out]
      }
      event #4 {
        n126 = event-data() -> ()  [unwired: 1 in, 6 out]
        n127 = disable-structure shown="Disabled" {
          frame #0 {
            n128 = Bundle("String"="no", "Value"=-1) -> (w206:cluster{"String":string, "Value":i32})  [unwired: 1 in]
            n129 = Bundle("String"="-", "Value"=-1) -> (w202:cluster{"String":string, "Value":i32})  [unwired: 1 in]
            n130 = Build Array(w206) -> (w207:cluster{"String":string, "Value":i32}[])
            n131 = Build Array(w202) -> (w201:cluster{"String":string, "Value":i32}[])
            n132 = for {
              tunnel: "Calib Container" -> [w219] mode=indexing
              shift-right: [w216] -> w205
              shift-left: w207 -> [w217]
              shift-right: [w211] -> w200
              shift-left: w201 -> [w212]
              i -> [w213]
              n133 = Unbundle By Name(w219) -> ("Ref Label"=w218:string, "Ref ID"=w214:i16)
              n134 = Greater Than 0?(x=w214) -> (x > 0?=w215:bool)
              n135 = Bundle("Ref Label"=w218, w213) -> (w210:cluster{"Ref Label":string, i32})  [unwired: 1 in]
              n136 = case shown="True" w215 {
                tunnel: w217 -> [w220 w223]
                tunnel: [w220 w222] -> w216
                tunnel: w210 -> [_ w221]
                frame #0 {
                }
                frame #1 {
                  n137 = Build Array (concatenate)(w223, w221) -> (w222:cluster{"Ref Label":string, "Value":i32}[])
                }
              }
              n138 = Build Array (concatenate)(w212, w210) -> (w211:cluster{"Ref Label":string, "Value":i32}[])
            }
            n139 = property on="Property Node" class="Ring (strict)"("StringsAndValues[]"=w205) -> ()  [unwired: 2 in, 2 out]
            n140 = property class="Ring (strict)"("StringsAndValues[]"=w200) -> ()  [unwired: 2 in, 2 out]
          }
          frame #1 {
          }
        }
      }
      event #5 {
        n141 = event-data() -> ()  [unwired: 1 in, 6 out]
        n142 = local read "ziCalib"() -> (w224:T6)
        n143 = Write to Binary File(data=w224, 5:FALSE ("prepend array or string size? (T)"), 9:T9."big-endian, network order" ("byte order (0:big-endian, network order)")) -> (refnum out=w226:refnum<file>)  [unwired: 3 in, 2 out]
        n144 = Close File(refnum=w226) -> ()  [unwired: 1 in, 2 out]
      }
      event #6 {
        n145 = event-data() -> ()  [unwired: 1 in, 6 out]
        n146 = disable-structure shown="Disabled" {
          frame #0 {
            n147 = Index Array() -> (element=w241)  [unwired: 2 in]
            n148 = Unbundle By Name(w241) -> ("Meas_Z"=w240)
            n149 = Divide(x=180.0, y=3.141592653589793) -> (x/y=w235:dbl)
            n150 = Index Array(array=w240, index (col) #1=0 ("disabled index (col)")) -> (element #1=w232, element #2=w233, element #3=w234)  [unwired: 5 in]
            n151 = control-ref of="Calibration R (Ohm)"() -> (w231:refnum<vi>)
            n152 = Multiply(x=w234, y=w235) -> (x*y=w236:dbl)
            n153 = Bundle(w232, w233) -> (w230:cluster{void, void})  [unwired: 1 in]
            n154 = Bundle(w232, w236) -> (w228:cluster{void, dbl})  [unwired: 1 in]
            n155 = property class="XYGraph (strict)"(reference=w231, "Value"=w230) -> ()  [unwired: 1 in, 2 out]
            n156 = control-ref of="Calibration Theta (deg)"() -> (w229:refnum<vi>)
            n157 = property class="XYGraph (strict)"(reference=w229, "Value"=w228) -> ()  [unwired: 1 in, 2 out]
          }
          frame #1 {
          }
        }
      }
      event #7 {
        n158 = event-data() -> ()  [unwired: 1 in, 6 out]
        n159 = Open/Create/Replace File() -> (refnum out=w244:refnum<file>)  [unwired: 6 in, 2 out]
        n160 = Read from Binary File(5:T6 {"Time Stamp"=timestamp(0 s since 1904-01-01), "Calib Model"=enum."Invalid", "ModelCoeffs"=[], "Meas (F,Z0,...,Zn)"=[]} ("ziCalib"), 9:T9."big-endian, network order" ("byte order (0:big-endian, network order)"), 10:1 ("count"), 11:w244) -> (2:w245:T6[], 3:w246:refnum<file>)  [unwired: 2 in, 2 out]
        n161 = Close File(refnum=w246) -> ()  [unwired: 1 in, 2 out]
        n162 = Index Array(array=w245) -> (element=w243:T6)  [unwired: 1 in]
        n163 = local write "ziCalib"(w243) -> ()
      }
      event #8 {
        # "Saves Conductivity"
        n164 = event-data() -> ()  [unwired: 1 in, 6 out]
        n165 = local read "Vz: Theta"() -> (w250:T2)
        n166 = local read "Phase(I) (deg)"() -> (w263:cluster{"Output":dbl[], dbl[]})
        n167 = local read "R (ohm)"() -> (w266:cluster{"Output":dbl[], dbl[]})
        n168 = local read "Vz: Amp"() -> (w252:T2)
        n169 = local read "Iz (Arms)"() -> (w262:cluster{"Output":dbl[], dbl[]})
        n170 = local read "C (F)"() -> (w267:cluster{"Output":dbl[], dbl[]})
        n171 = Unbundle(w266) -> (w253:dbl[])  [unwired: 1 out]
        n172 = Index Array(array=w250) -> (element=w249:T4)  [unwired: 1 in]
        n173 = Index Array(array=w252) -> (element=w251:T4)  [unwired: 1 in]
        n174 = Unbundle(w262) -> (w259:dbl[])  [unwired: 1 out]
        n175 = Unbundle(w263) -> (w258:dbl[])  [unwired: 1 out]
        n176 = Unbundle(w251) -> (w261:dbl[])  [unwired: 1 out]
        n177 = Unbundle(w249) -> (w260:dbl[])  [unwired: 1 out]
        n178 = Reciprocal(x=w253) -> (1/x=w254:dbl[])
        n179 = Unbundle(w267) -> ("Output"=w265:dbl[], w264:dbl[])
        n180 = Build Array(w265, w264, w254, w261, w260, w259, w258) -> (w256:dbl[][])
        n181 = call-poly <vilib>:"Write To Spreadsheet File.vi"("transpose? (no:F)"=TRUE, "format (%.3f)"="%8g", "2D data"=w256) -> ()  [unwired: 5 in, 1 out]
      }
      event #9 {
        n182 = event-data() -> ("NewVal"=w268:i16)  [unwired: 1 in, 5 out]
        n183 = Decrement(x=w268) -> (x-1=w270:i16)
        n184 = Greater Than 0?(x=w268) -> (x > 0?=w269:bool)
        n185 = case shown="True" w269 {
          tunnel: w270 -> [_ w278]
          frame #0 {
            w271 = FALSE ("Visible")
            n186 = property on="R (Ohms)" class="DigNum (strict)"("Visible"=w271) -> ()  [unwired: 2 in, 2 out]
            n187 = property on="Ref 2" class="DigNum (strict)"("Visible"=w271) -> ()  [unwired: 2 in, 2 out]
            n188 = property on="Ref 3" class="DigNum (strict)"("Visible"=w271) -> ()  [unwired: 2 in, 2 out]
          }
          frame #1 {
            n189 = disable-structure shown="Enabled" {
              disable-tunnel: w278 -> [w291 _]
              disable-tunnel: [w284 "R (ohm)"] -> w277
              disable-tunnel: [w283 _] -> w276
              disable-tunnel: [w282 "C (F)"] -> w275
              disable-tunnel: [w281 w293] -> w274
              disable-tunnel: [w280 _] -> w273
              disable-tunnel: [w279 w293] -> w272
              frame #0 {
                n190 = local read "cal_types"() -> (w288:cluster{string[], bool[]}[])
                n191 = Index Array(array=w288, index=w291) -> (element=w287:cluster{string[], bool[]})
                n192 = Unbundle(w287) -> (w286:string[], w285:bool[])
                n193 = Index Array(array=w286, index #1=0 ("index")) -> (element #1=w284:string, element #2=w282:string, element #3=w283:string)  [unwired: 2 in]
                n194 = Index Array(array=w285, index #1=0 ("index")) -> (element #1=w281:bool, element #2=w279:bool, element #3=w280:bool)  [unwired: 2 in]
              }
              frame #1 {
                w293 = TRUE
              }
            }
            n195 = property on="R (Ohms)" class="DigNum (strict)"("Caption.Text"=w277, "Visible"=w274) -> ()  [unwired: 2 in, 2 out]
            n196 = property on="Ref 2" class="DigNum (strict)"("Caption.Text"=w275, "Visible"=w272) -> ()  [unwired: 2 in, 2 out]
            n197 = property on="Ref 3" class="DigNum (strict)"("Caption.Text"=w276, "Visible"=w273) -> ()  [unwired: 2 in, 2 out]
          }
        }
      }
      event #10 {
        n198 = event-data() -> ()  [unwired: 1 in, 8 out]
        n199 = control-ref of="Raw Theta"() -> (w307:refnum<vi>)
        n200 = control-ref of="C (F)"() -> (w310:refnum<vi>)
        n201 = control-ref of="R (ohm)"() -> (w309:refnum<vi>)
        n202 = control-ref of="Raw Voltage"() -> (w308:refnum<vi>)
        n203 = control-ref of="Phase(I) (deg)"() -> (w306:refnum<vi>)
        n204 = control-ref of="Iz (Arms)"() -> (w305:refnum<vi>)
        n205 = control-ref of="Vz: Theta"() -> (w304:refnum<vi>)
        n206 = control-ref of="Vz: Amp"() -> (w303:refnum<vi>)
        n207 = Build Array(w310, w309) -> (w302:refnum<vi>[])
        n208 = Build Array(w308, w307) -> (w301:refnum<vi>[])
        n209 = Build Array(w304, w303) -> (w299:refnum<vi>[])
        n210 = Build Array(w306, w305) -> (w300:refnum<vi>[])
        n211 = control-ref of="Calibration R (Ohm)"() -> (w296:refnum<vi>)
        n212 = control-ref of="Calibration Theta (deg)"() -> (w297:refnum<vi>)
        n213 = Build Array(w297, w296) -> (w295:refnum<vi>[])
        n214 = Build Array(w302, w301, w300, w299, w295) -> (w298:refnum<vi>[][])
        n215 = for {
          tunnel: w298 -> [w313] mode=indexing
          n216 = Index Array(array=w313) -> (element #1=w312:refnum<vi>, element #2=w311:refnum<vi>)  [unwired: 2 in]
          n217 = property class="XYGraph"(reference=w312) -> ("XScale.Range"=w314:T11)  [unwired: 1 in, 2 out]
          n218 = property class="XYGraph"(reference=w311, "XScale.Range"=w314) -> ()  [unwired: 1 in, 2 out]
        }
      }
      event #11 {
        n219 = event-data() -> ()  [unwired: 1 in, 6 out]
        n220 = local read "Iz Mode"() -> (w315:u16)
        n221 = case shown="1" w315 {
          frame #0 {
            n222 = property on="Shunt Resistor" class="DigNum (strict)"("Visible"=FALSE) -> ()  [unwired: 2 in, 2 out]
            n223 = property on="Voltage Gain" class="DigNum (strict)"("Visible"=FALSE) -> ()  [unwired: 2 in, 2 out]
            n224 = property on="Iz ZCtrl" class="Ring (strict)"("Caption.Text"="TA ZCtrl", "Visible"=TRUE) -> ()  [unwired: 2 in, 2 out]
            n225 = property on="PreampChannel" class="Ring (strict)"("Caption.Text"="TA Channel", "Visible"=TRUE) -> ()  [unwired: 2 in, 2 out]
          }
          frame #1 {
            n226 = property on="Shunt Resistor" class="DigNum (strict)"("Visible"=FALSE) -> ()  [unwired: 2 in, 2 out]
            n227 = property on="Voltage Gain" class="DigNum (strict)"("Visible"=FALSE) -> ()  [unwired: 2 in, 2 out]
            n228 = property on="Iz ZCtrl" class="Ring (strict)"("Caption.Text"="CA ZCtrl", "Visible"=TRUE) -> ()  [unwired: 2 in, 2 out]
            n229 = property on="PreampChannel" class="Ring (strict)"("Caption.Text"=" ", "Visible"=FALSE) -> ()  [unwired: 2 in, 2 out]
          }
          frame #2 {
            n230 = property on="Shunt Resistor" class="DigNum (strict)"("Visible"=FALSE) -> ()  [unwired: 2 in, 2 out]
            n231 = property on="Voltage Gain" class="DigNum (strict)"("Visible"=FALSE) -> ()  [unwired: 2 in, 2 out]
            n232 = property on="Iz ZCtrl" class="Ring (strict)"("Caption.Text"=" ", "Visible"=FALSE) -> ()  [unwired: 2 in, 2 out]
            n233 = property on="PreampChannel" class="Ring (strict)"("Caption.Text"=" ", "Visible"=FALSE) -> ()  [unwired: 2 in, 2 out]
          }
          frame #3 {
            n234 = property on="Shunt Resistor" class="DigNum (strict)"("Visible"=TRUE) -> ()  [unwired: 2 in, 2 out]
            n235 = property on="Voltage Gain" class="DigNum (strict)"("Visible"=TRUE) -> ()  [unwired: 2 in, 2 out]
            n236 = property on="Iz ZCtrl" class="Ring (strict)"("Value"="Shunt Resistor", "Visible"=FALSE) -> ()  [unwired: 2 in, 2 out]
            n237 = property on="PreampChannel" class="Ring (strict)"("Value"="Voltage Gain", "Visible"=FALSE) -> ()  [unwired: 2 in, 2 out]
          }
        }
      }
      event #12 {
        n238 = event-data() -> ()  [unwired: 1 in, 6 out]
        n239 = local read "Vz Mode"() -> (w340:u16)
        n240 = case shown="1" w340 {
          frame #0 {
            n241 = property on="Voltage Gain 2" class="DigNum (strict)"("Visible"=FALSE) -> ()  [unwired: 2 in, 2 out]
            n242 = property on="Vz ZCtrl" class="Ring (strict)"("Caption.Text"="Output Cha", "Visible"=TRUE) -> ()  [unwired: 2 in, 2 out]
          }
          frame #1 {
            n243 = property on="Voltage Gain 2" class="DigNum (strict)"("Visible"=TRUE) -> ()  [unwired: 2 in, 2 out]
            n244 = property on="Vz ZCtrl" class="Ring (strict)"("Value"="Voltage Gain 2", "Visible"=FALSE) -> ()  [unwired: 2 in, 2 out]
          }
          frame #2 {
            n245 = property on="Voltage Gain 2" class="DigNum (strict)"("Visible"=FALSE) -> ()  [unwired: 2 in, 2 out]
            n246 = property on="Vz ZCtrl" class="Ring (strict)"("Caption.Text"="CA ZCtrl", "Visible"=TRUE) -> ()  [unwired: 2 in, 2 out]
          }
        }
      }
    }
  }
  n247 = call <instrlib>:"ziClose.vi"("Error In"=w8, "Handle In"=w9) -> ()  [unwired: 2 in, 2 out]
